vi "r3_Pick&Place_module_chip_second.vi"() -> ()   [LabVIEW 2016]
uses:
  Classes/Controllers/I-O/Copy of NI-DAQ Folder/NI-DAQ.lvclass
  D:/INTT/V1/Classes/Controllers/I-O/Copy of I-O Folder/I-O.lvclass
  Classes/Controllers/Dispenser/Copy of Ultimus V2 Folder/Ultimus V2.lvclass
  <vilib>/Analysis/coordinate.llb/2D Cartesian Coordinate Rotation (Scalar).vi
  <vilib>/Utility/file.llb/Read Delimited Spreadsheet (DBL).vi
  <vilib>/Utility/file.llb/Write Delimited Spreadsheet (DBL).vi
  Classes/Controllers/Motion/Copy of Motion Folder/Motion.lvclass
  Classes/Controllers/Camera/Copy of Controller Folder/Controller.lvclass
  <vilib>/Analysis/NI_AALPro.lvlib
  Classes/Controllers/I-O/Copy of I-O Folder/I-O.lvclass
panel:
  in  "offset":dbl[](array[numeric])
  out "air pressure indecator":i32
  in  "glue deposit group":i32=4
  in  "Ultimus Pressure":i16=20
  in  "Values":bool[](array[boolean])=[FALSE, FALSE]
  out "vacuum on?":bool[](array[boolean])
  out "Array 2":dbl[][](array[numeric])
  out "Measured PickupTool position":dbl[][](array[numeric])
  in  "sampel vacuum":i32[](array[numeric])=[15, 19]
  in  "VacChannel for sample":i32=1
  in  "TrayVaccum":bool
  in  "check height? 2":bool
  in  "check height?":bool
  out "Needle parking position":dbl[](array[numeric])
  out "GlueBox":dbl[][](array[numeric])
  out "appended array":dbl[][](array[numeric])
  in  "chip placement height compensation":dbl=-0.47 format="%#_13g"
  out "Sample on HDI":dbl[][](array[numeric]) format="%#_8g"
  in  "Sensor A/B":bool
  out "Gantry current position":dbl[](array[numeric])
  in  "READ Position":bool
  in  "Needle Height Compenstation\n(glue gap)":dbl=0.34
  in  "Needle Alignment":bool
  in  "Parking position":dbl[](array[numeric])=[625.0, 625.0, 0.0, 0.01]
  in  "GOTO":bool
  in  "Default Pickup Tool Position":dbl[][](array[numeric])=[[153.043, 779.997, 54.962, 0.0365632], [153.043, 779.997, 54.962, 0.0365632]]
  in  "Number of Chips/Sensors \nto be assembled":i32=1
  in  "Default HDI alignment \nmark position":dbl[](array[numeric])=[292.437, 991.477, 79.3487, -0.011805]
  in  "Default HDI size":dbl[](array[numeric])=[24.3371, 231.337, -0.0132064, -0.000194865]
  out "# of tasks excuted":i32
  out "Chips on tray position":dbl[][](array[numeric])
  out "measured HDI size":dbl[](array[numeric])
  in  "Chip tray":dbl[](array[numeric])=[465.031, 710.639, 69.8028, 0.00407755]
  out "Sample position \non HDI":dbl[][](array[numeric])
  in  "Inititalize":bool
  in  "Pick and place":bool
  in  "Deposit Glue":bool
  in  "Measure Pickup Tools":bool
  in  "Measure Samples on tray":bool
  out "default chip and sensor position w.r.t. 1st mark":dbl[][](array[numeric])
  in  "Assembly Type":bool=TRUE
  in  "Stop":bool
  in  "Measure HDI":bool
  out "Measure HDI top-left":dbl[](array[numeric])
  # "Sensor Tray \nVacuum Channel"
  # "Chips"
  # "Sensor 0.3 -> 200 micron glue thickness\nChips 0.34-> 150 micron glue thickness"
  # "Sensors"
  # "Sensor B short"
  # "Sensors B\n(Short)"
  # "Sensors A\n(Long)"
  # "Chips : -0.47-> 60 micron height gap\n               -0.5 -> 90 micron"
  # "Sensor A long"
  # "ACTIONS"
  # "2"
  # "HDI infomation"
  # "chips use channel 0, 2\nsensors use channel 0, 1"
  # "sensor height 69.8471\nchip height 84.693"
  # "Pick and Place"
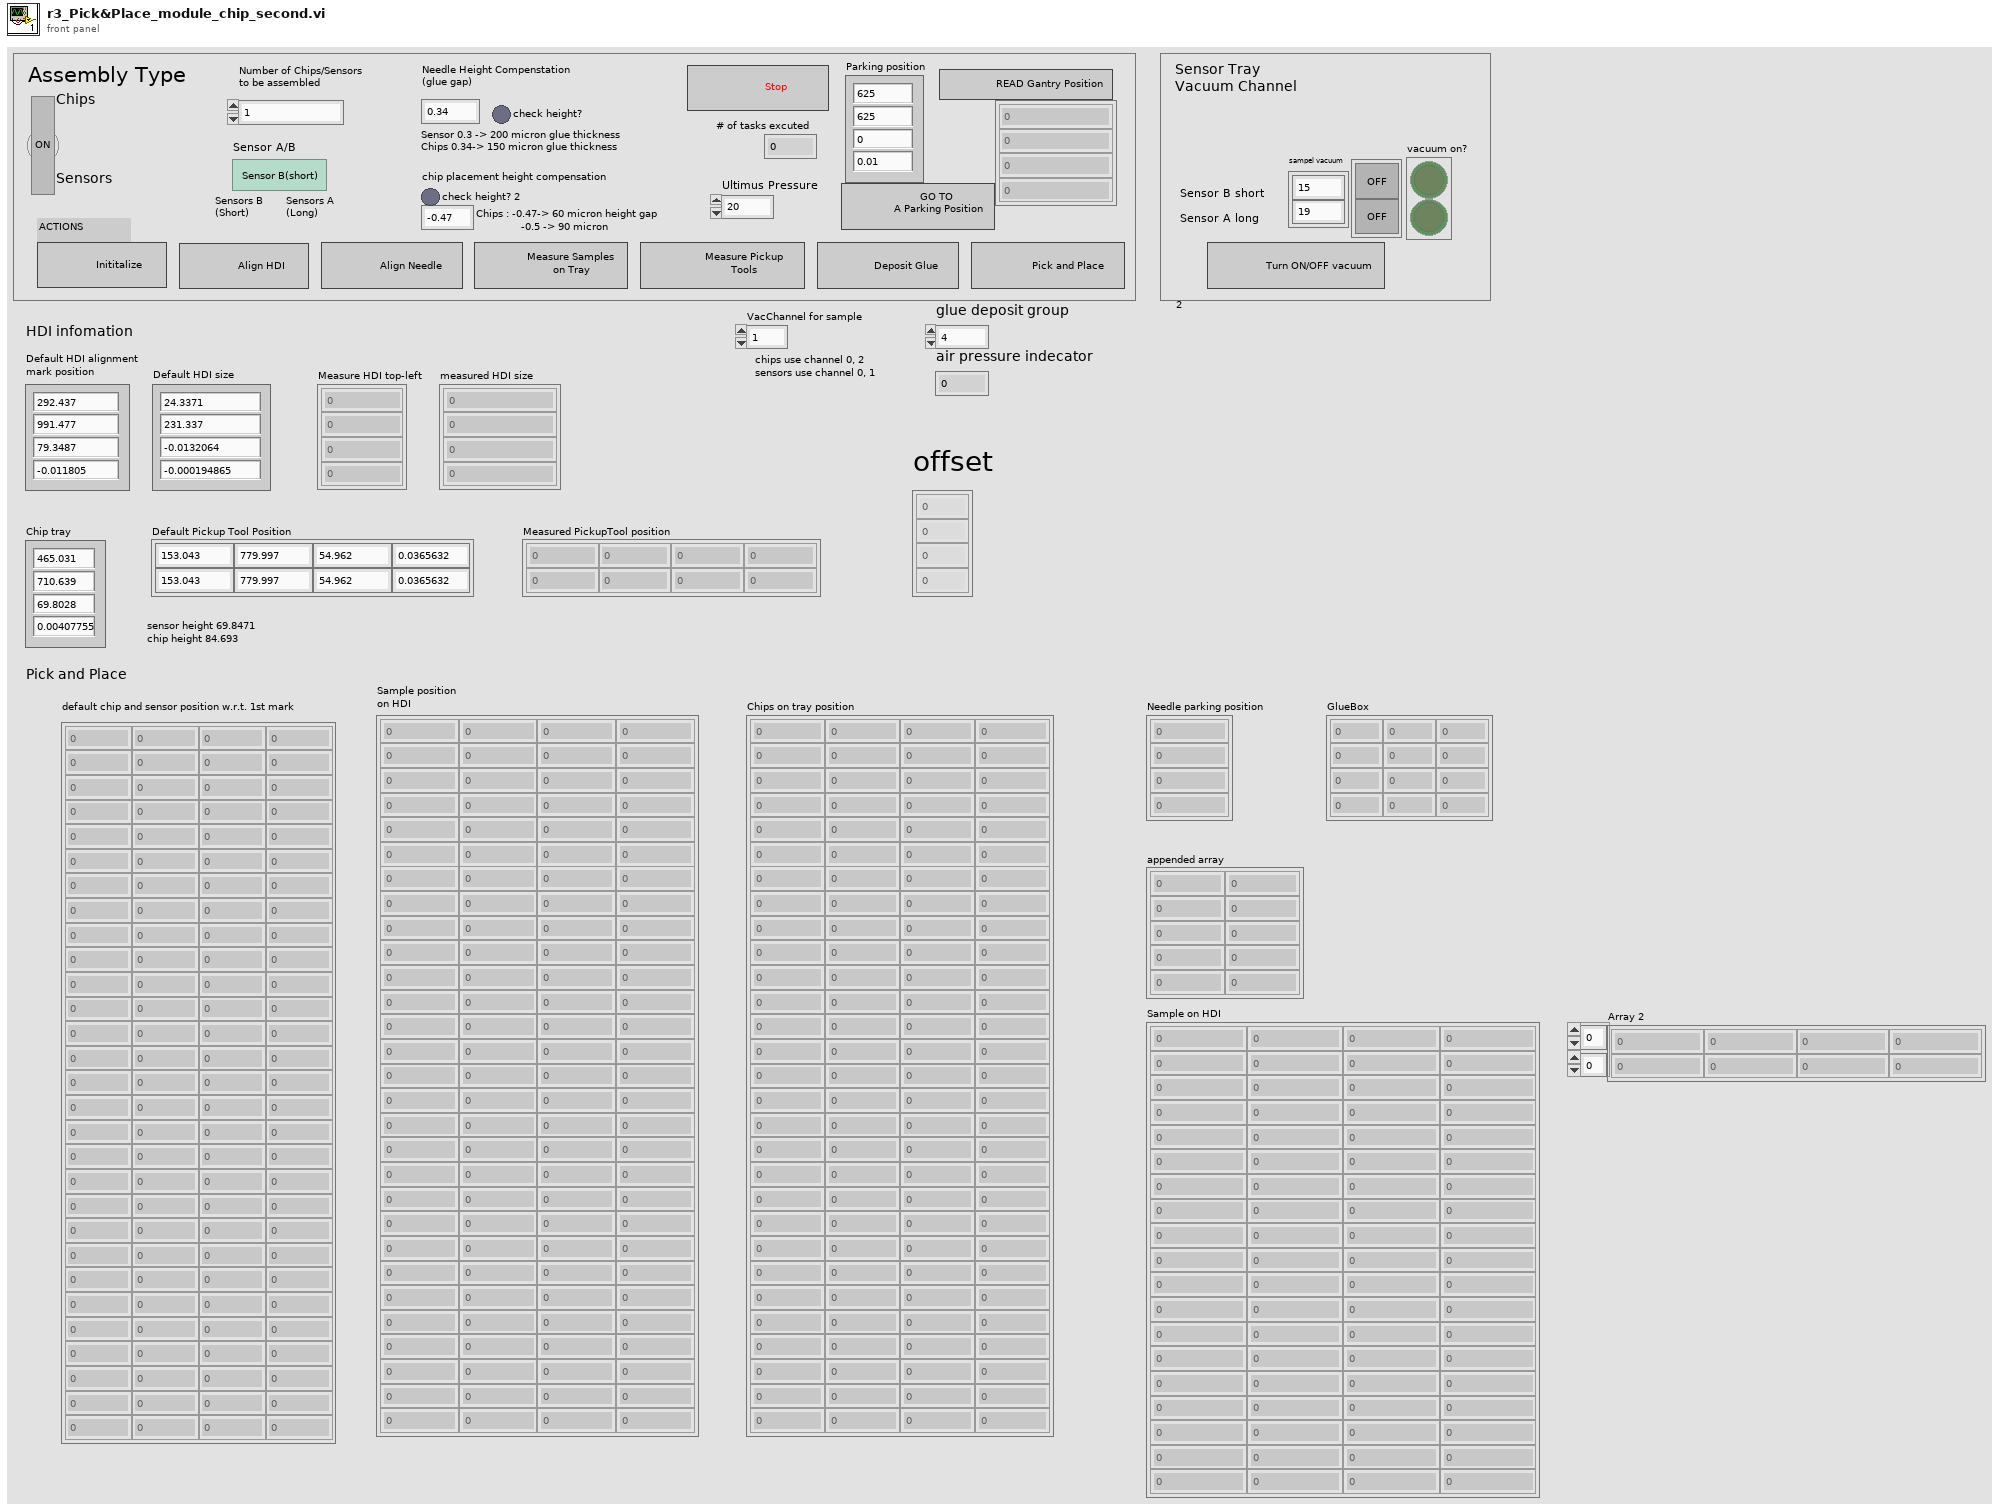
[diagram p1: front panel]
types:
  T1 = typedef "Controller.lvclass/Controllers.ctl" = cluster{"Copy of Motion.lvclass":refnum<class "Motion.lvclass">, "Copy of I-O.lvclass":refnum<class "I-O.lvclass">, "Copy of Dispenser.lvclass":refnum<class "Dispenser.lvclass">}
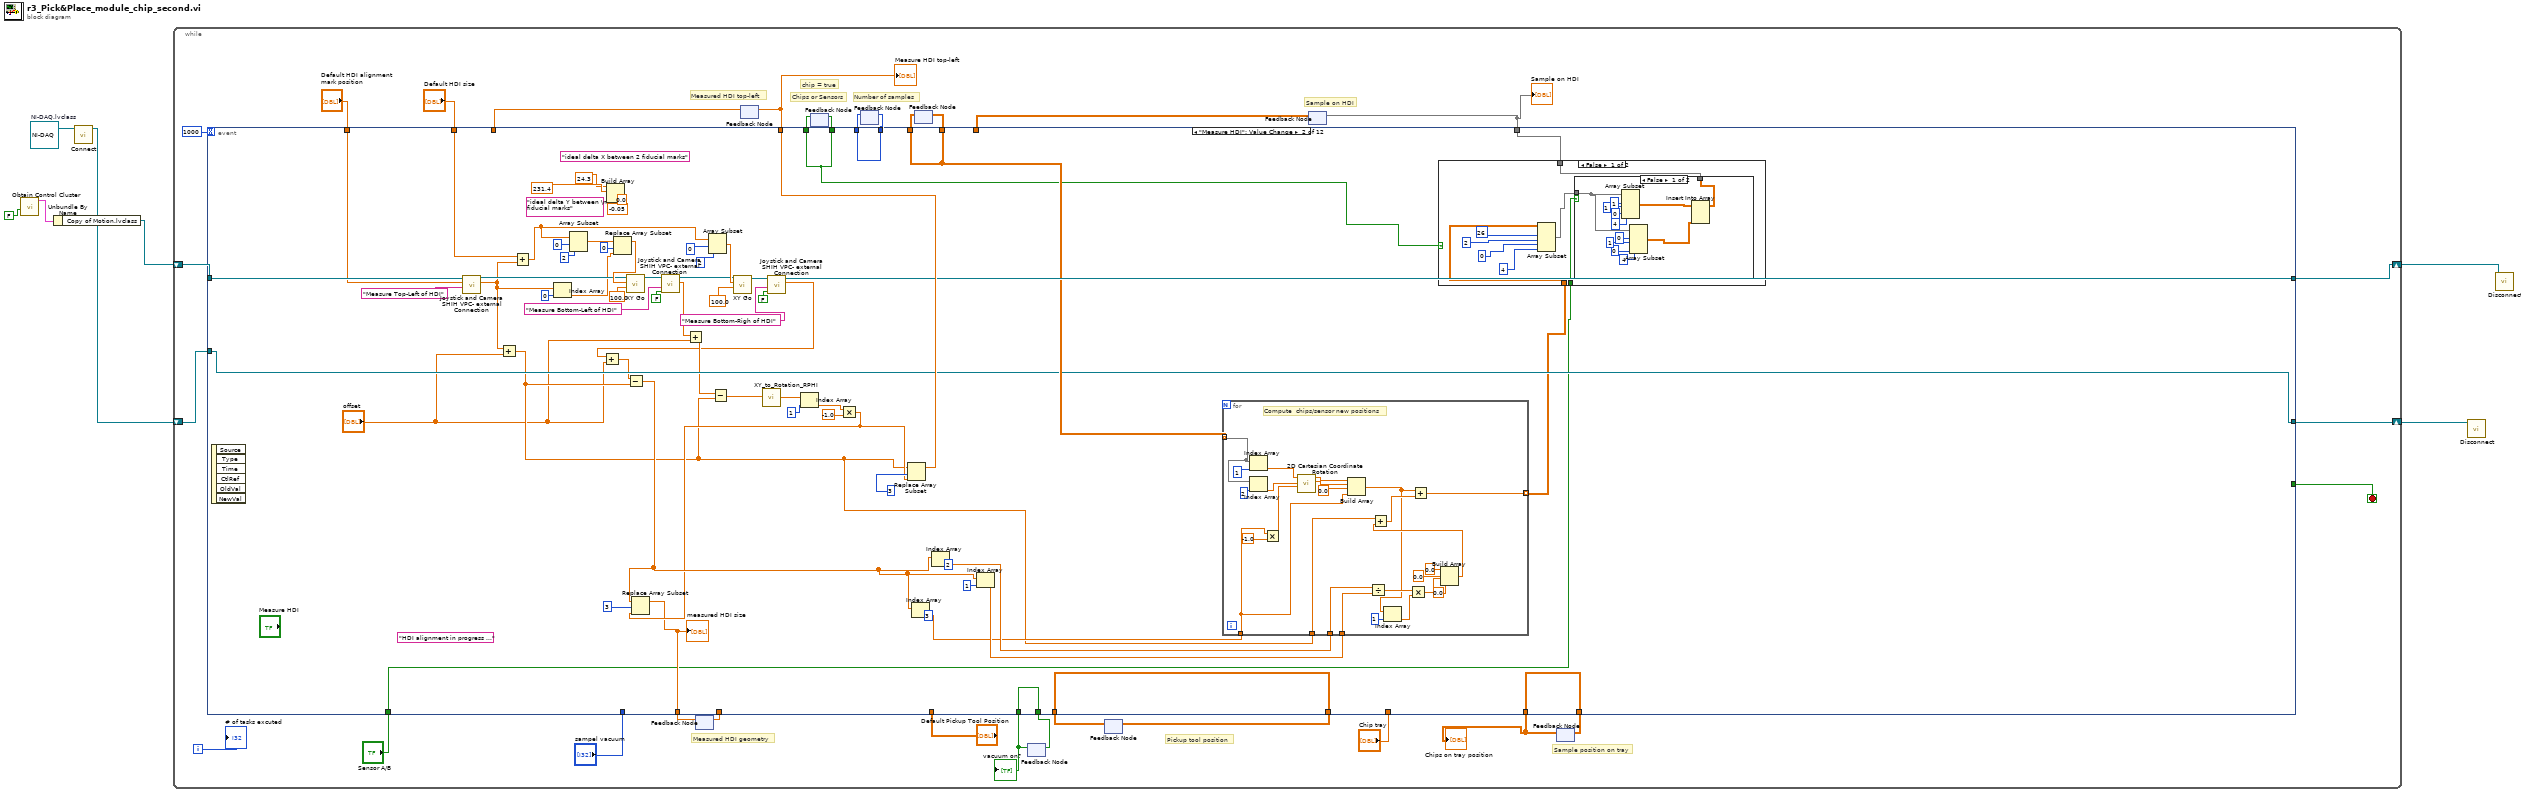
[diagram p0: block diagram]
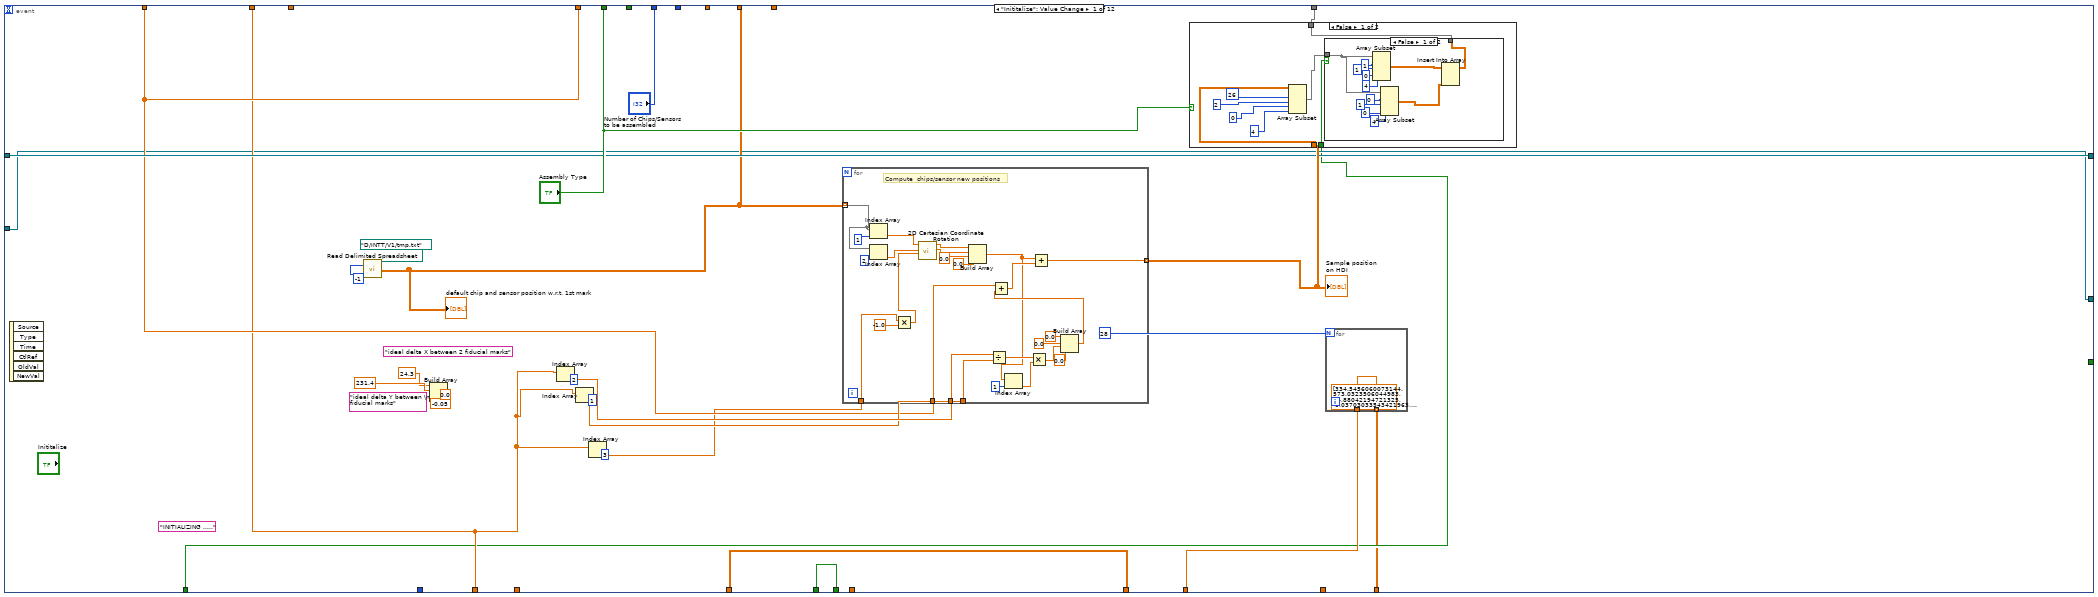
[diagram p2: hidden frame]
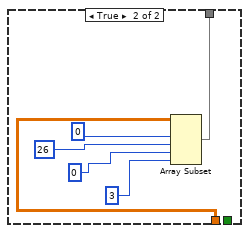
[diagram p4: hidden frame]
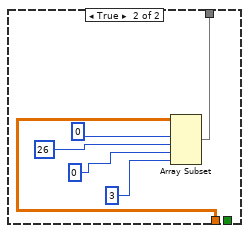
[diagram p6: hidden frame]
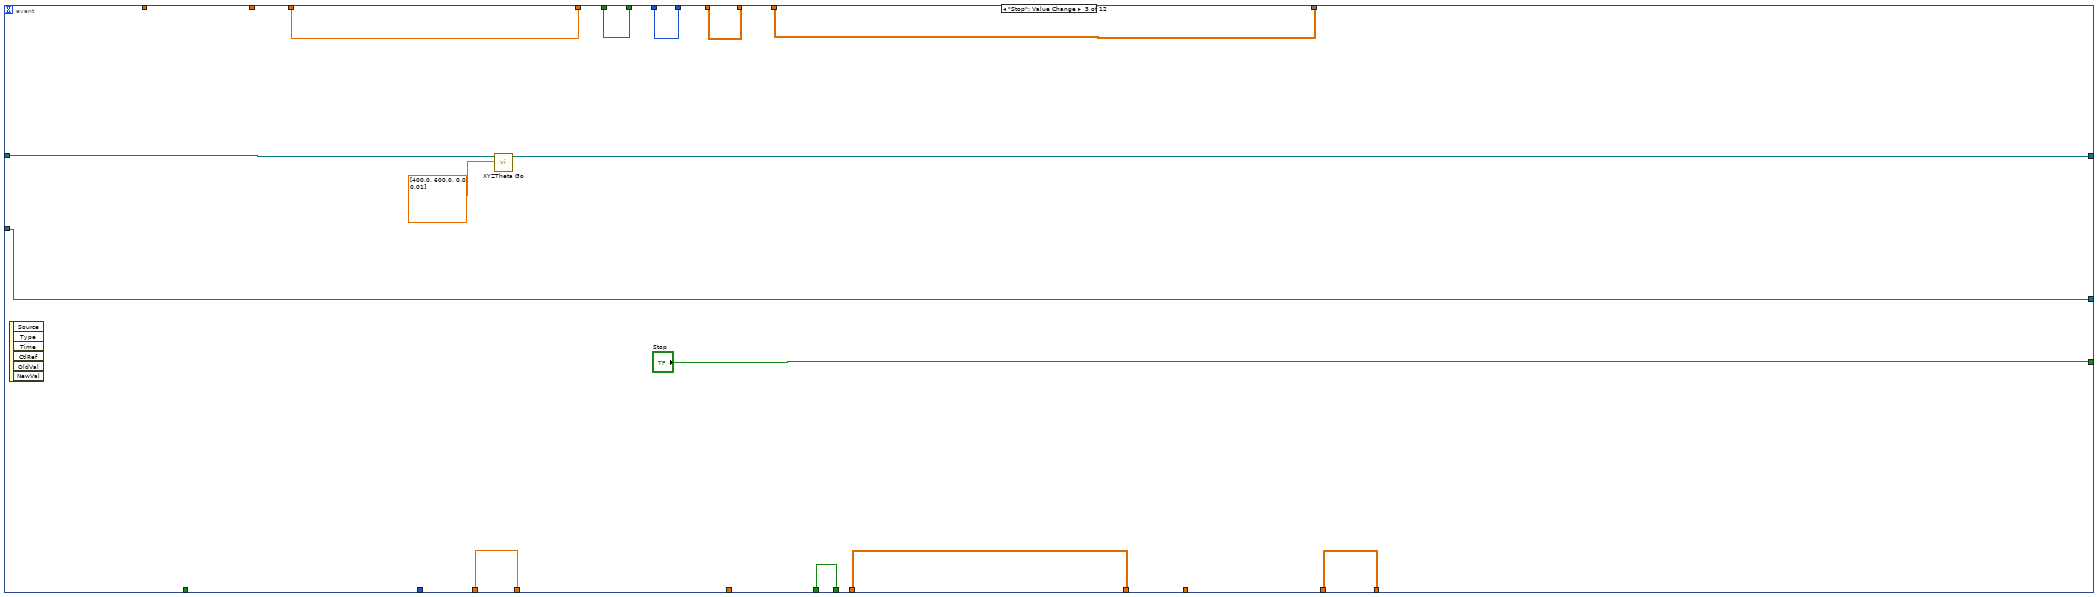
[diagram p7: hidden frame]
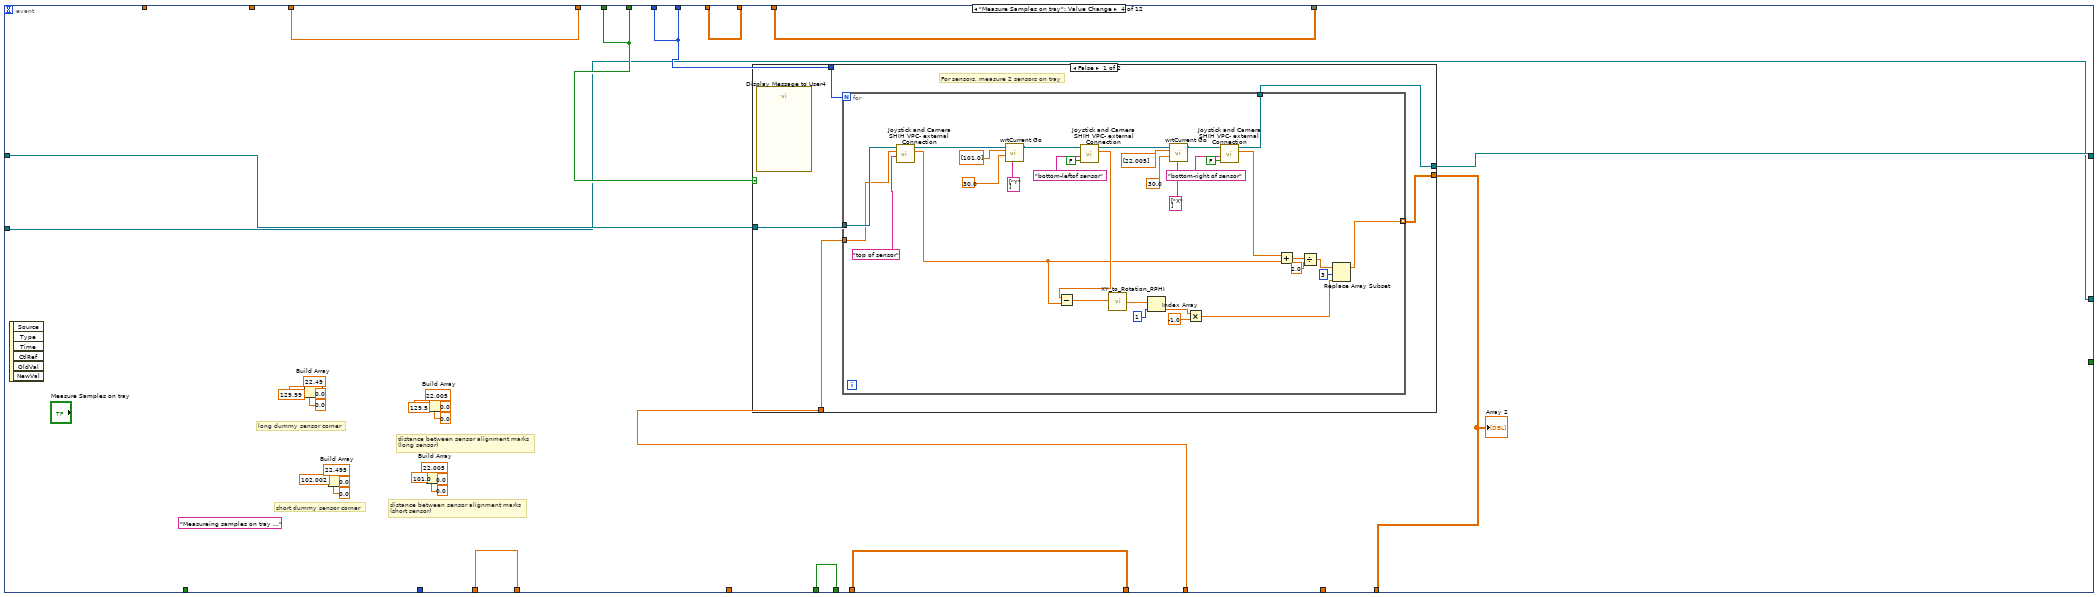
[diagram p8: hidden frame]
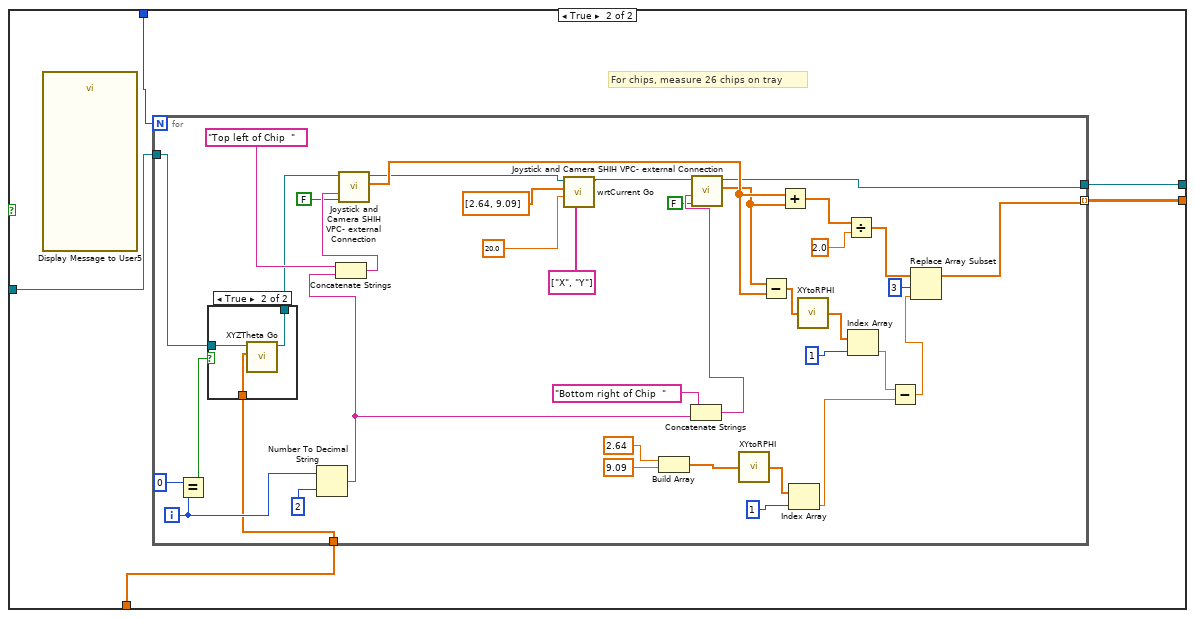
[diagram p9: hidden frame]
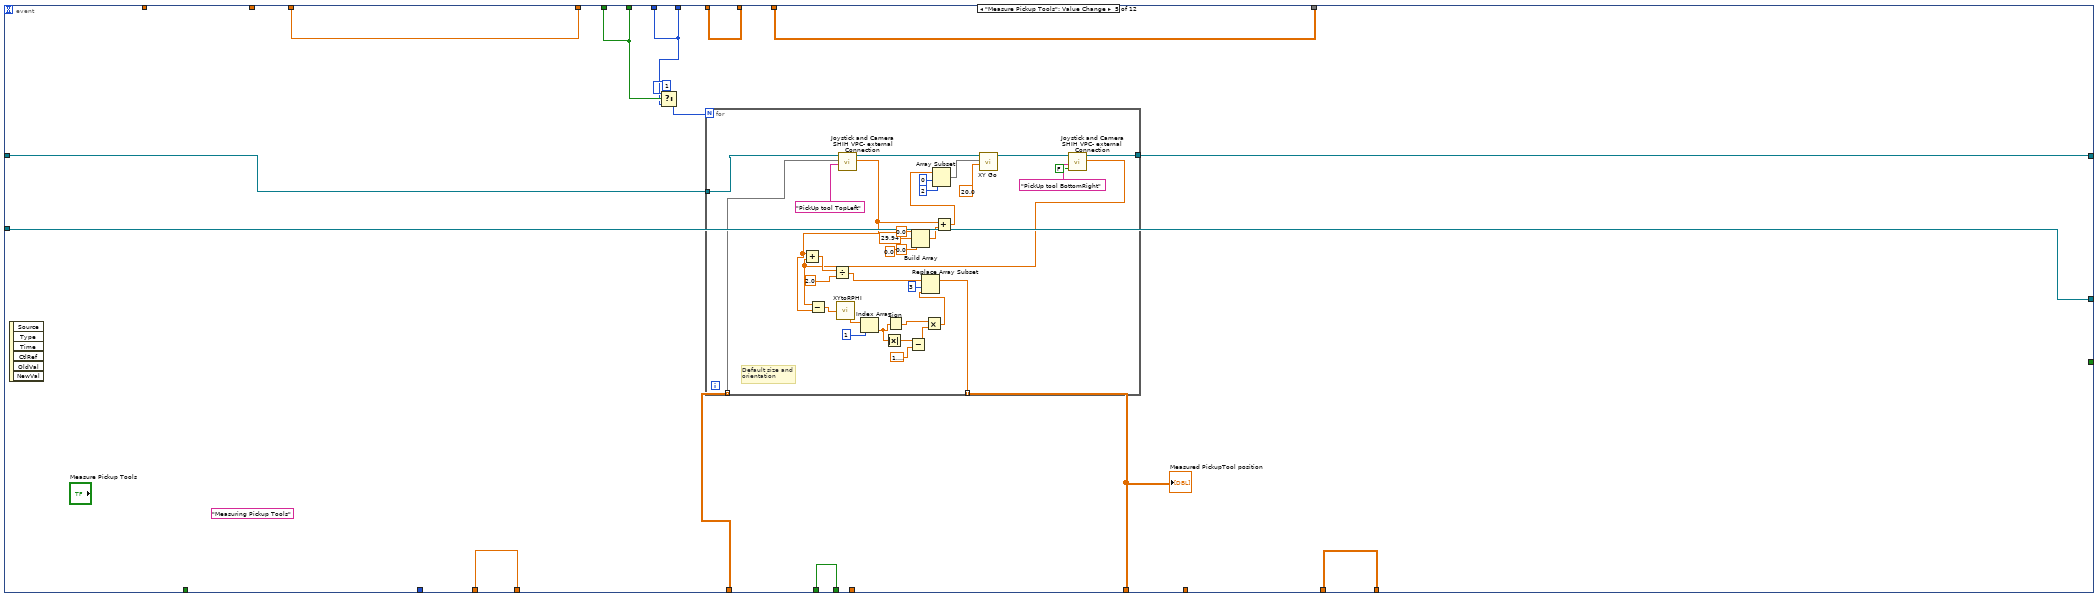
[diagram p11: hidden frame]
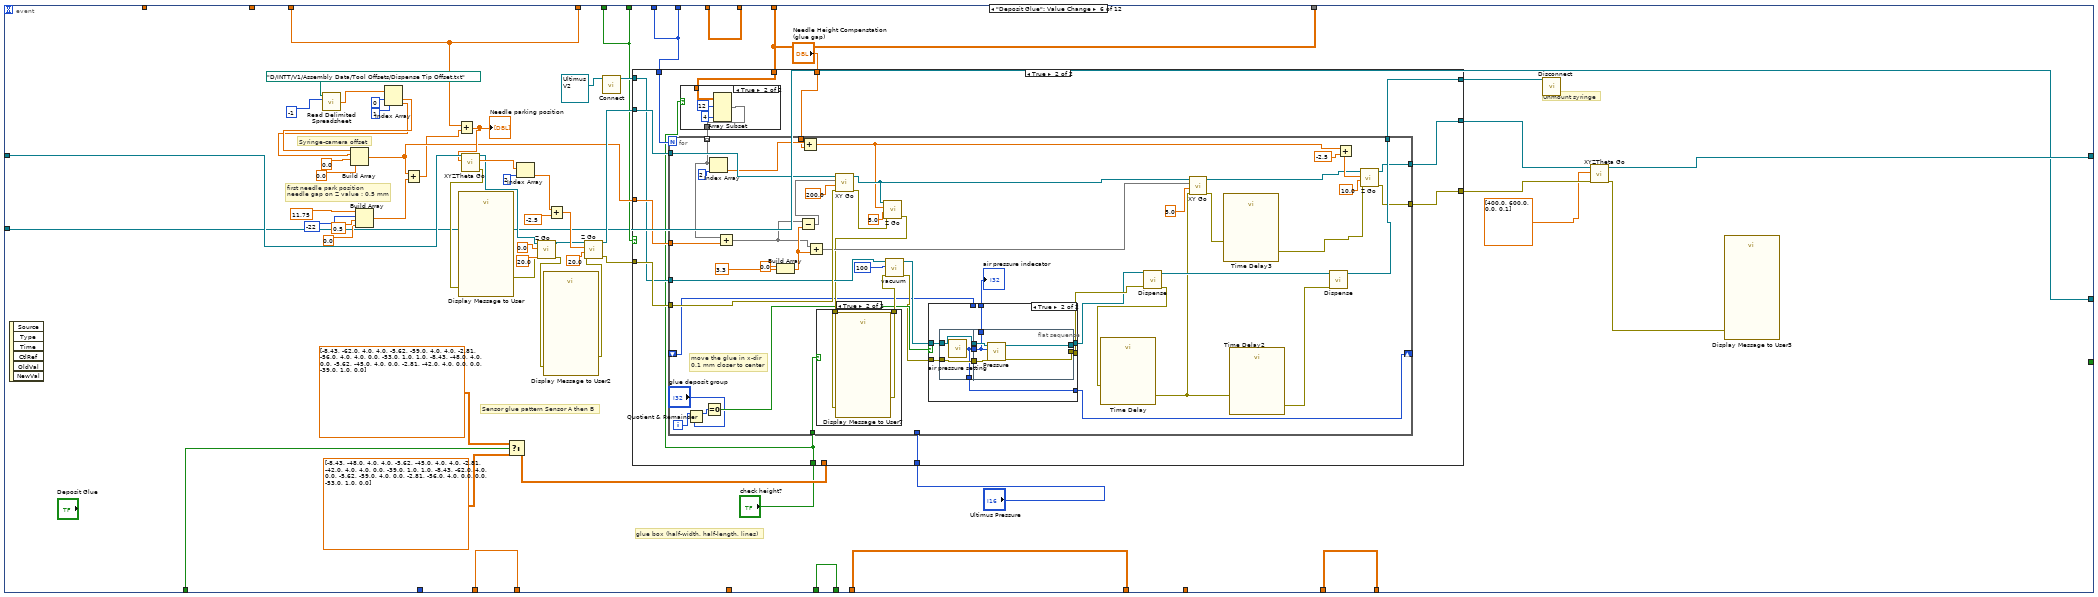
[diagram p12: hidden frame]
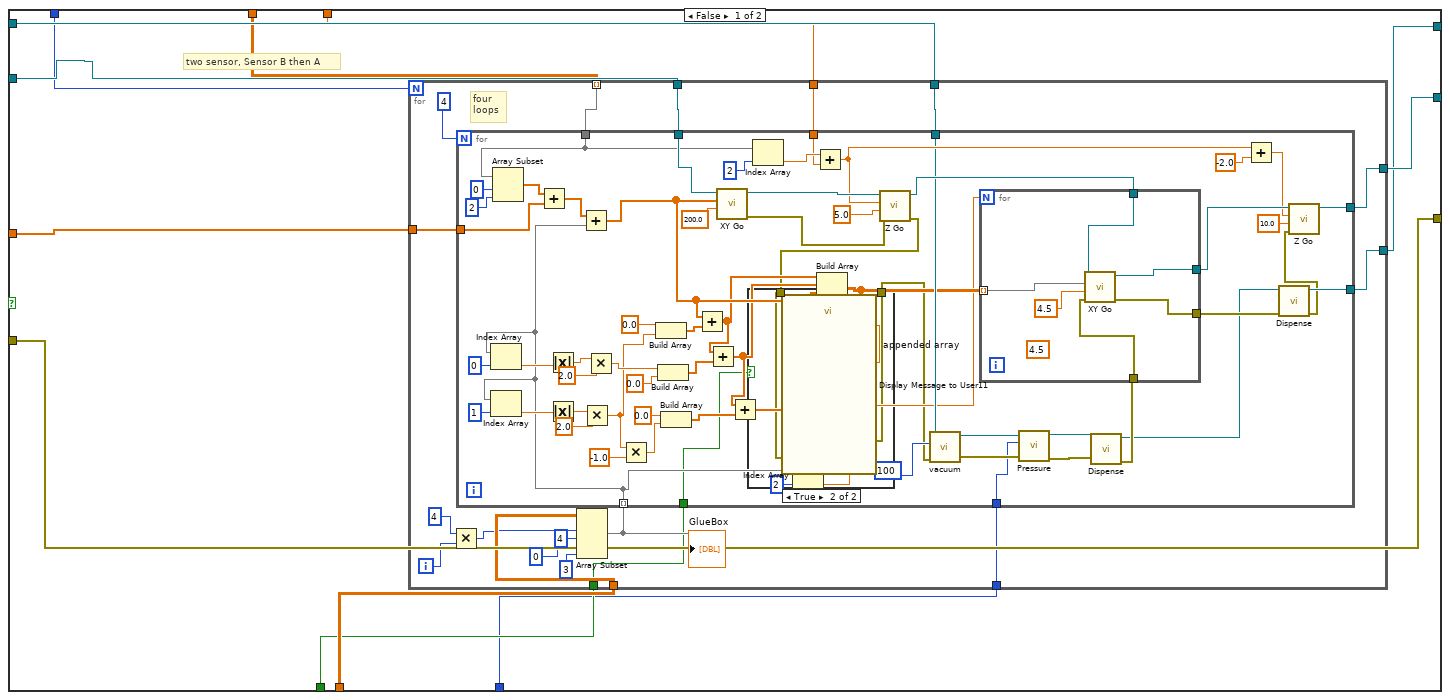
[diagram p13: hidden frame]
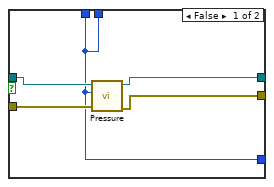
[diagram p16: hidden frame]
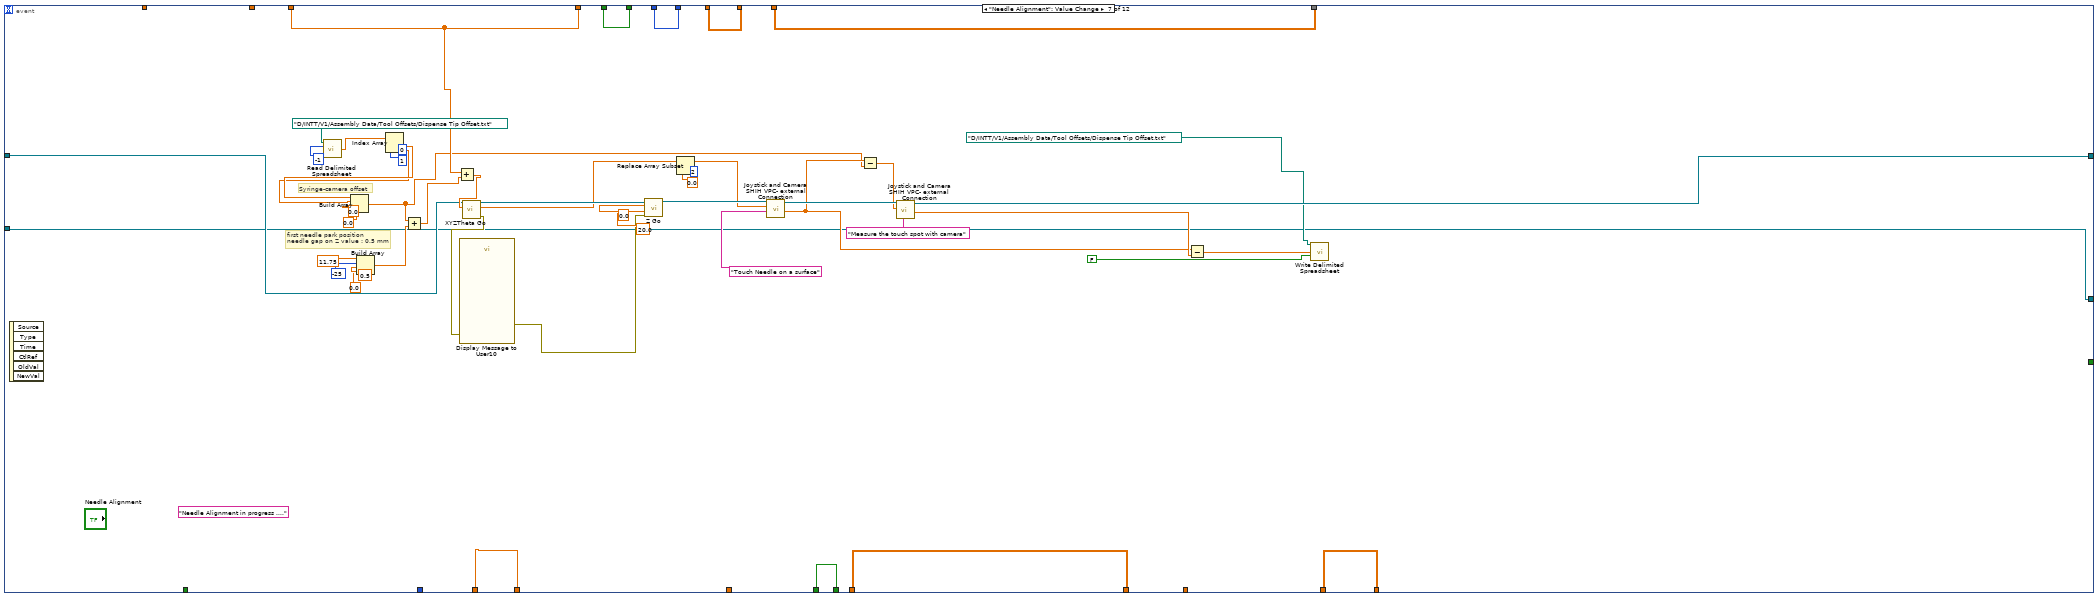
[diagram p18: hidden frame]
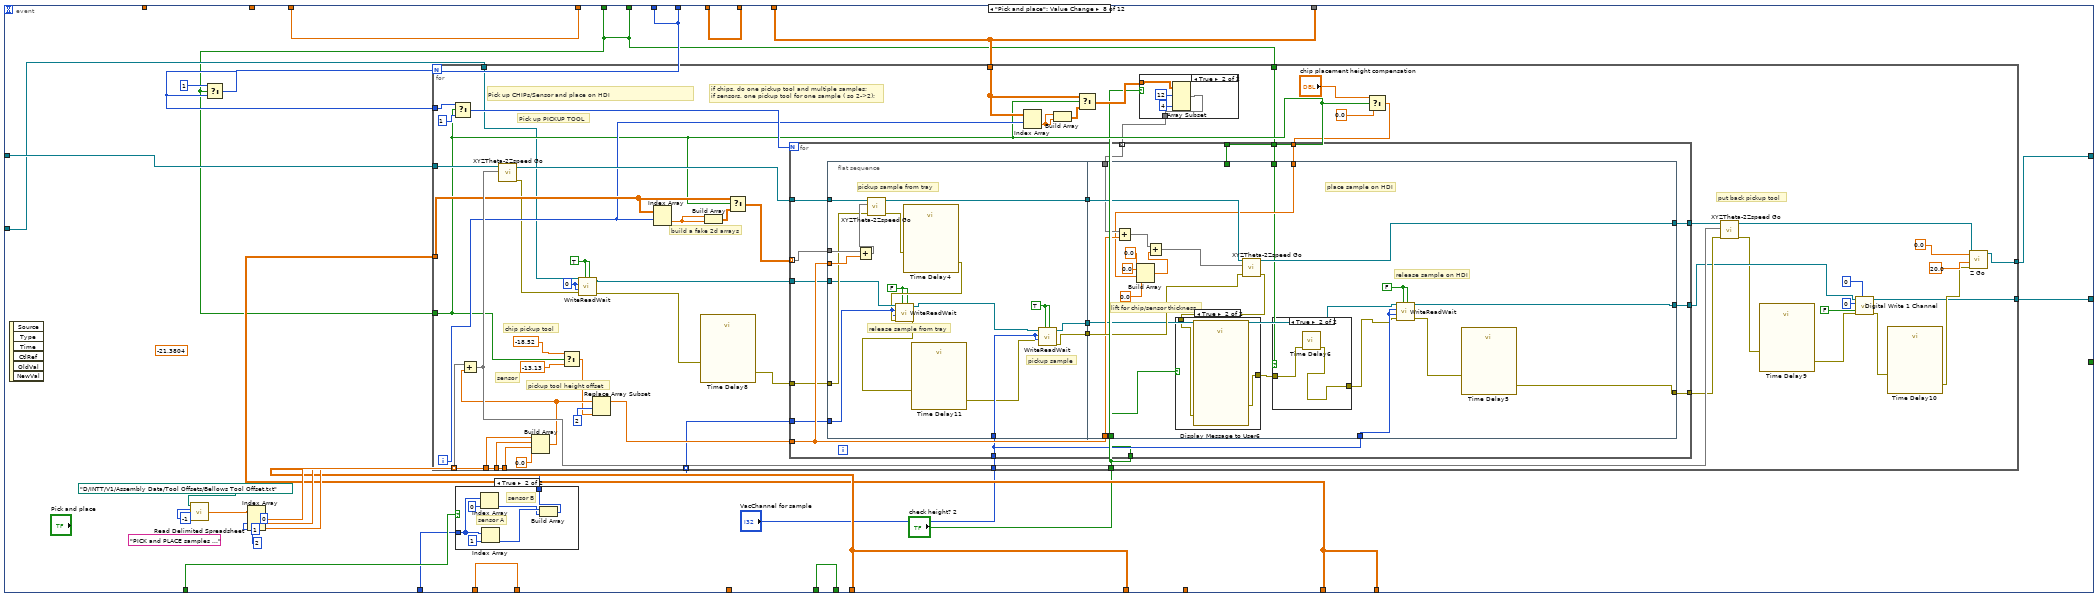
[diagram p19: hidden frame]
diagram:
  w3 = refnum<class "NI-DAQ.lvclass"> refnum  # NI-DAQ.lvclass
  n1 = call "Obtain Control Cluster.vi"("I/O"=FALSE) -> ("Control Out"=w7:T1)  [unwired: 10 in]
  n2 = Unbundle By Name(w7) -> ("Copy of Motion.lvclass"=w5:refnum<class "Motion.lvclass">)
  n3 = call-dynamic "Connect.vi"("NI-DAQ in"=w3) -> ("NI-DAQ out"=w2:refnum<class "NI-DAQ.lvclass">)  [unwired: 9 in, 1 out]
  n4 = while {
    shift-right: [w26] -> w4
    shift-left: w5 -> [w38]
    shift-right: [w13] -> w1
    shift-left: w2 -> [w14]
    i -> [w25]
    stop <- w37 stop-if-true
    # "chip = true"
    # "Pickup tool position"
    # "Chips or Sensors"
    # "Number of samples"
    # "Measured HDI geometry"
    # "Sample position on tray"
    # "Measured HDI top-left"
    # "Sample on HDI"
    n5 = feedback #1() -> (w33:dbl[])  [unwired: 1 in]
    n6 = feedback #2() -> (w35:dbl[])  [unwired: 1 in]
    n7 = feedback #3() -> (w30:bool)  [unwired: 1 in]
    n8 = feedback #4() -> (w24:i32)  [unwired: 1 in]
    n9 = feedback #5() -> (w19:dbl[][])  [unwired: 1 in]
    n10 = feedback #6() -> (w10:bool[])  [unwired: 1 in]
    n11 = feedback #7() -> (w27:dbl[][])  [unwired: 1 in]
    n12 = feedback #8() -> (w32:dbl[][])  [unwired: 1 in]
    n13 = feedback #9() -> (w16:dbl[][])  [unwired: 1 in]
    "Chips on tray position" <- w16
    n14 = event shown="[1] \"Measure HDI\": Value Change" {
      selector: _ -> [_ _ _ _ _ _ _ _ _ _ _ _]
      dyn-events: _ -> [_ _ _ _ _ _ _ _ _ _ _ _]
      timeout: 1000 -> [_ _ _ _ _ _ _ _ _ _ _ _]
      tunnel: w38 -> [w52 w183 w249 w278 w376 w445 w681 w737 w878 w900 w924 w926]
      tunnel: [_ _ "Stop" _ _ _ _ _ _ _ _ _] -> w37
      tunnel: [w49 w181 w242 w272 w367 w426 w689 w721 w887 w894 w920 w937] -> w36
      tunnel: w35 -> [_ _ w242 w272 w367 w426 w689 w721 w887 w894 w920 w937]
      tunnel: ["Assembly Type" w129 w246 w276 w372 w429 w688 w711 w886 w895 w921 w936] -> w31
      tunnel: [w45 w133 w241 w271 w366 w422 w684 w720 w882 w893 w919 w930] -> w34
      tunnel: w33 -> [_ _ w241 w271 w366 w422 w684 w720 w882 w893 w919 w930]
      tunnel: [w40 w130 w243 w273 w369 w428 w685 w726 w883 w898 w923 w933] -> w8
      tunnel: w32 -> [_ _ w243 w273 w369 w428 w685 w726 w883 w898 w923 w933]
      tunnel: w30 -> [_ w129 w246 w276 w372 w429 w688 w711 w886 w895 w921 w936]
      tunnel: w24 -> [_ w172 w245 w275 w371 w427 w687 w723 w885 w896 w916 w935]
      tunnel: [w39 w170 w239 w252 w365 w424 w682 w724 w880 w891 w917 w932] -> w29
      tunnel: w16 -> [_ w170 w239 _ w365 w424 w682 w724 w880 w891 w917 w932]
      tunnel: [w48 w171 w240 w270 w375 w423 w683 w725 w881 w892 w918 w931] -> w28
      tunnel: w27 -> [_ w171 w240 w270 _ w423 w683 w725 w881 w892 w918 w931]
      tunnel: [w52 w180 w247 w277 w374 w430 w673 w727 w877 w899 w924 w926] -> w26
      tunnel: ["Number of Chips/Sensors \nto be assembled" w172 w245 w275 w371 w427 w687 w723 w885 w896 w916 w935] -> w23
      tunnel: "Default HDI alignment \nmark position" -> [w49 w179 _ _ _ _ _ _ _ _ _ _]
      tunnel: "Default HDI size" -> [w45 w178 _ _ _ _ _ _ _ _ _ _]
      tunnel: [w50 w173 w244 w274 w368 w421 w686 w722 w884 w897 w922 w934] -> w20
      tunnel: w19 -> [_ w173 w244 w274 w368 w421 w686 w722 w884 w897 w922 w934]
      tunnel: "Default Pickup Tool Position" -> [w48 _ _ _ w370 _ _ _ _ _ _ _]
      tunnel: "Chip tray" -> [w47 _ _ w269 _ _ _ _ _ _ _ _]
      tunnel: "Sensor A/B" -> [w42 w128 _ _ _ w420 _ w719 _ _ _ _]
      tunnel: w14 -> [w43 w132 w237 w251 w364 w414 w664 w716 w879 w889 w915 w927]
      tunnel: [w43 w132 w237 w251 w364 w414 w664 w717 w879 w889 w901 w925] -> w13
      tunnel: "sampel vacuum" -> [_ _ _ _ _ _ _ w713 _ _ w903 w928]
      tunnel: [w41 w131 w236 w250 w363 w413 w663 w712 w875 w888 w902 w929] -> w11
      tunnel: w10 -> [w41 w131 w236 w250 w363 w413 w663 w712 w875 w888 w902 _]
      event "Inititalize": Value Change {
        (unwired) dbl[][] [[334.5456060073144, 573.0323506044983, 84.88042194721325, -0.03703033543421963], [348.7343172517964, 572.8622513715641, 84.88042161151989, 0.002496633181773955], [362.2570314501057, 572.9994237111084, 84.87348419133077, 0.0034316271147138977], [374.6597880882888, 573.1847541366935, 84.85760352984227, -0.00879928913304795], [388.2847032482186, 573.1649677768512, 84.84172357788742, -0.026054726433181852], [334.1328739355822, 593.938164573938, 84.85715223326392, 0.0033385186776999642], [348.32260344605317, 593.1627350557167, 84.85715229429908, 0.032527677556001944], [361.94845426967004, 593.1988990556995, 84.85715231337257, 0.010856722342177383], [375.3711307391728, 592.862734170051, 84.81179255805122, 0.023593691294119035], [388.0023391138823, 592.7263595201845, 84.81179247794259, -0.025867399820654446], [333.741332819156, 613.4501439838673, 84.86893968673877, 0.012458442710573392], [347.4966613938597, 613.1815273693476, 84.84113487130284, 0.02669962172184226], [360.982501589219, 613.368579091193, 84.84113464623572, -0.018470295852746066], [333.329425210144, 634.0016681075332, 84.84113694649815, -0.011509836209115054], [347.60697621578583, 633.6458142671074, 84.84113655739904, -0.014006699863984284], [362.03055194039933, 633.3683242670324, 84.84113543587804, 0.008503358353721735], [374.6669884842355, 633.6776673973038, 84.82931378598124, -0.012163463061963586], [388.449715198344, 634.0661620162508, 84.81749059876144, -0.029966589814424793], [334.6459562288677, 653.6797245247765, 84.85127519810308, -0.010927379491059153], [348.144539580008, 653.7156084768662, 84.88505952278655, -0.012269636914733706], [361.33508542794345, 653.7223221455167, 84.84332432319749, -0.0225512602477429], [374.2287534347454, 653.8981636020831, 84.87276718319089, 0.0007662059738136051], [387.0483029791335, 653.6404602098912, 84.83290343994173, 0.01982829778783901], [334.77129192493265, 669.5351603609607, 84.8979373024785, 0.03923574774306138], [347.17815774254836, 669.4879675513143, 84.9183079020849, 0.003793410140892961], [361.84116966674696, 669.9123563355322, 84.87756716463502, 0.02903318407151878]] ("Chips on tray position")
        (unwired) "INITIALIZING ....." ("String")
        (unwired) "ideal delta Y between \n2 fiducial marks"
        (unwired) "ideal delta X between 2 fiducial marks"
        n15 = event-data() -> ()  [unwired: 1 in, 6 out]
        n16 = call-poly <vilib>:"Read Delimited Spreadsheet.vi"("file path (dialog if empty)"=path "D:/INTT/V1/tmp.txt", "number of rows (all:-1)"=-1) -> ("all rows"=w50:dbl[][])  [unwired: 8 in, 5 out]
        "default chip and sensor position w.r.t. 1st mark" <- w50
        n17 = Build Array(24.3 ("y"), 231.4 ("y"), 0.0 ("element"), -0.05 ("element")) -> ()  [unwired: 1 out]
        n18 = Index Array(array=w45, index=2) -> (element=w61:dbl)
        n19 = Index Array(array=w45, index=1) -> (element=w60:dbl)
        n20 = Index Array(array=w45, index=3) -> (element=w44:dbl)
        n21 = for {
          tunnel: w50 -> [w112] mode=indexing
          tunnel: w44 -> [w95]
          tunnel: w49 -> [w104]
          tunnel: [w111] -> w54 mode=indexing
          tunnel: w61 -> [w110]
          tunnel: w60 -> [w101]
          # "Compute  chips/sensor new positions"
          n22 = Index Array(array=w112, index=1) -> (element=w116:dbl)
          n23 = Index Array(array=w112, index=2) -> (element=w115:dbl)
          n24 = Multiply(x=w95, y=-1.0) -> (x*y=w96:dbl)
          n25 = call-poly <vilib>:"2D Cartesian Coordinate Rotation.vi"("theta"=w96, "y"=w115, "x"=w116) -> ("y out"=w118:dbl, "x out"=w117:dbl)  [unwired: 6 in, 1 out]
          n26 = Build Array(w117, w118, 0.0 ("element"), 0.0 ("element")) -> (w98:dbl[])
          n27 = Divide(x=w110, y=w101) -> (x/y=w109:dbl)
          n28 = Index Array(array=w98, index=1) -> (element=w99:dbl)
          n29 = Multiply(x=w109, y=w99) -> (x*y=w105:dbl)
          n30 = Build Array(0.0 ("element"), 0.0 ("element"), w105, 0.0 ("element")) -> (w103:dbl[])
          n31 = Add(x=w104, y=w103) -> (x+y=w102:dbl[])
          n32 = Add(x=w98, y=w102) -> (x+y=w111:dbl[])
        }
        "Sample position \non HDI" <- w54
        n33 = case shown="False" "Assembly Type" {
          tunnel: w54 -> [w69 w89]
          tunnel: [w67 w87] -> w40
          tunnel: w42 -> [w66 _]
          frame False {
            n34 = Array Subset(array=w69, index (row)=26 ("index"), length (row)=2 ("length"), index (col)=0, length (col)=4 ("length")) -> (w68:dbl[][])
            n35 = case shown="False" w66 {
              tunnel: w68 -> [w77 w86]
              tunnel: [w74 w86] -> w67
              frame False {
                n36 = Array Subset(array=w77, index (row)=1 ("index"), length (row)=1 ("length"), index (col)=0 ("index"), length (col)=4 ("length")) -> (w76:dbl[][])
                n37 = Array Subset(array=w77, index (row)=0 ("index"), length (row)=1 ("length"), index (col)=0 ("index"), length (col)=4 ("length")) -> (w75:dbl[][])
                n38 = Insert Into Array(array=w76, new element=w75) -> (w74:dbl[][])  [unwired: 2 in]
              }
              frame True {
              }
            }
          }
          frame True {
            n39 = Array Subset(array=w89, index (row)=0 ("index"), length (row)=26 ("length"), index (col)=0, length (col)=3 ("length")) -> (w87:dbl[][])
          }
        }
        n40 = for {
          N: 28 -> [_]
          tunnel: w47 -> [w93]
          tunnel: [w93] -> w39 mode=indexing
        }
      }
      event "Measure HDI": Value Change {
        (unwired) "ideal delta Y between \n2 fiducial marks"
        (unwired) "ideal delta X between 2 fiducial marks"
        (unwired) "HDI alignment in progress ..." ("String")
        n41 = event-data() -> ()  [unwired: 1 in, 6 out]
        n42 = call "Joystick and Camera SHIH VPC- external Connection.vi"("Motion in"=w183, "XYZTheta"=w179, "Measurement Point"="Measure Top-Left of HDI") -> ("Motion out"=w148:refnum<class "Motion.lvclass">, "Sum"=w126:dbl[])  [unwired: 4 in, 2 out]
        n43 = Add(x=w126, y="offset") -> (x+y=w125:dbl[])
        n44 = Add(x=w178, y=w126) -> (x+y=w152:dbl[])
        n45 = Index Array(array=w126, index=0) -> (element=w139:dbl)
        n46 = Array Subset(array=w152, index=0, length=2) -> (w151:dbl[])
        n47 = Build Array(24.3 ("y"), 231.4 ("y"), 0.0 ("element"), -0.05 ("element")) -> ()  [unwired: 1 out]
        n48 = Replace Array Subset(array=w151, new element=w139, index=0) -> (w149:dbl[])
        n49 = call-dynamic "XY Go.vi"("Speed"=100.0, "XY"=w149, "Motion in"=w148) -> ("Motion out"=w156:refnum<class "Motion.lvclass">)  [unwired: 7 in, 1 out]
        n50 = call "Joystick and Camera SHIH VPC- external Connection.vi"("Motion in"=w156, "Measurement Point"="Measure Bottom-Left of HDI", "Inital GO"=FALSE) -> ("Motion out"=w147:refnum<class "Motion.lvclass">, "Sum"=w124:dbl[])  [unwired: 4 in, 2 out]
        n51 = Add(x=w124, y="offset") -> (x+y=w123:dbl[])
        n52 = Array Subset(array=w152, index=0, length=2) -> (w162:dbl[])
        n53 = Subtract(x=w123, y=w125) -> (x-y=w146:dbl[])
        n54 = call-dynamic "XY Go.vi"("Speed"=100.0, "XY"=w162, "Motion in"=w147) -> ("Motion out"=w166:refnum<class "Motion.lvclass">)  [unwired: 7 in, 1 out]
        n55 = call "XY_to_Rotation_RPHI.vi"("X-Y"=w146) -> ("r-phi"=w142:dbl[])
        n56 = call "Joystick and Camera SHIH VPC- external Connection.vi"("Motion in"=w166, "Measurement Point"="Measure Bottom-Righ of HDI", "Inital GO"=FALSE) -> ("Motion out"=w180:refnum<class "Motion.lvclass">, "Sum"=w122:dbl[])  [unwired: 4 in, 2 out]
        n57 = Add(x=w122, y="offset") -> (x+y=w121:dbl[])
        n58 = Subtract(x=w121, y=w125) -> (x-y=w136:dbl[])
        n59 = Index Array(array=w142, index=1) -> (element=w137:dbl)
        n60 = Multiply(x=w137, y=-1.0) -> (x*y=w134:dbl)
        n61 = Replace Array Subset(array=w136, new element=w134, index=3) -> (w133:dbl[])
        "measured HDI size" <- w133
        n62 = Replace Array Subset(array=w125, new element=w134, index=3) -> (w181:dbl[])
        n63 = Index Array(array=w136, index=3) -> (element=w168:dbl)
        n64 = Index Array(array=w136, index=2) -> (element=w175:dbl)
        n65 = Index Array(array=w136, index=1) -> (element=w174:dbl)
        n66 = for {
          tunnel: w173 -> [w228] mode=indexing
          tunnel: w168 -> [w213]
          tunnel: w125 -> [w221]
          tunnel: w175 -> [w227]
          tunnel: w174 -> [w218]
          tunnel: [w211] -> w127 mode=indexing
          # "Compute  chips/sensor new positions"
          n67 = Index Array(array=w228, index=1) -> (element=w232:dbl)
          n68 = Index Array(array=w228, index=2) -> (element=w231:dbl)
          n69 = Multiply(x=w213, y=-1.0) -> (x*y=w212:dbl)
          n70 = call-poly <vilib>:"2D Cartesian Coordinate Rotation.vi"("theta"=w212, "y"=w231, "x"=w232) -> ("y out"=w234:dbl, "x out"=w233:dbl)  [unwired: 6 in, 1 out]
          n71 = Build Array(w233, w234, 0.0 ("element"), w213) -> (w215:dbl[])
          n72 = Divide(x=w227, y=w218) -> (x/y=w226:dbl)
          n73 = Index Array(array=w215, index=1) -> (element=w216:dbl)
          n74 = Multiply(x=w226, y=w216) -> (x*y=w222:dbl)
          n75 = Build Array(0.0 ("element"), 0.0 ("element"), w222, 0.0 ("element")) -> (w220:dbl[])
          n76 = Add(x=w221, y=w220) -> (x+y=w219:dbl[])
          n77 = Add(x=w215, y=w219) -> (x+y=w211:dbl[])
        }
        n78 = case shown="False" w129 {
          tunnel: w127 -> [w187 w207]
          tunnel: [w185 w205] -> w130
          tunnel: w128 -> [w184 _]
          frame False {
            n79 = Array Subset(array=w187, index (row)=26 ("index"), length (row)=2 ("length"), index (col)=0, length (col)=4 ("length")) -> (w186:dbl[][])
            n80 = case shown="False" w184 {
              tunnel: w186 -> [w195 w204]
              tunnel: [w192 w204] -> w185
              frame False {
                n81 = Array Subset(array=w195, index (row)=1 ("index"), length (row)=1 ("length"), index (col)=0 ("index"), length (col)=4 ("length")) -> (w194:dbl[][])
                n82 = Array Subset(array=w195, index (row)=0 ("index"), length (row)=1 ("length"), index (col)=0 ("index"), length (col)=4 ("length")) -> (w193:dbl[][])
                n83 = Insert Into Array(array=w194, new element=w193) -> (w192:dbl[][])  [unwired: 2 in]
              }
              frame True {
              }
            }
          }
          frame True {
            n84 = Array Subset(array=w207, index (row)=0 ("index"), length (row)=26 ("length"), index (col)=0, length (col)=3 ("length")) -> (w205:dbl[][])
          }
        }
      }
      event "Stop": Value Change {
        n85 = event-data() -> ()  [unwired: 1 in, 6 out]
        n86 = call "XYZTheta Go.vi"("XYZTheta In"=dbl[] [400.0, 600.0, 0.0, 0.01], "Motion in"=w249) -> ("Motion out"=w247:refnum<class "Motion.lvclass">)  [unwired: 7 in, 2 out]
      }
      event "Measure Samples on tray": Value Change {
        (unwired) "Measureing samples on tray ..." ("String")
        # "long dummy sensor corner"
        # "short dummy sensor corner"
        # "distance between sensor alignment marks\n(short sensor)"
        # "distance between sensor alignment marks\n(long sensor)"
        n87 = event-data() -> ()  [unwired: 1 in, 6 out]
        n88 = Build Array(22.49 ("element"), 129.99 ("element"), 0.0 ("element"), 0.0 ("element")) -> ()  [unwired: 1 out]
        n89 = Build Array(22.495 ("element"), 102.002 ("element"), 0.0 ("element"), 0.0 ("element")) -> ()  [unwired: 1 out]
        n90 = Build Array(22.005 ("element"), 101.0 ("element"), 0.0 ("element"), 0.0 ("element")) -> ()  [unwired: 1 out]
        n91 = Build Array(22.005 ("element"), 129.5 ("element"), 0.0 ("element"), 0.0 ("element")) -> ()  [unwired: 1 out]
        n92 = case shown="False" w276 {
          tunnel: [w280 w320] -> w252
          tunnel: w278 -> [w283 w319]
          tunnel: [w279 w318] -> w277
          tunnel: w275 -> [w282 w317]
          tunnel: w269 -> [w281 w316]
          frame False {
            # "For sensors, measure 2 sensors on tray"
            n93 = call "Display Message to User4"() -> ()  [unwired: 10 in, 2 out]
            n94 = for {
              N: w282 -> [_]
              tunnel: w283 -> [w315]
              tunnel: [w312] -> w279
              tunnel: [w306] -> w280 mode=indexing
              tunnel: w281 -> [w305]
              n95 = call "Joystick and Camera SHIH VPC- external Connection.vi"("Motion in"=w315, "XYZTheta"=w305, "Measurement Point"="top of sensor") -> ("Motion out"=w287:refnum<class "Motion.lvclass">, "Sum"=w294:dbl[])  [unwired: 4 in, 2 out]
              n96 = call-dynamic "wrtCurrent Go.vi"("axis names"=string[] ["Y"], "Speed"=30.0, "distances"=dbl[] [101.0], "Motion in"=w287) -> ("Motion out"=w286:refnum<class "Motion.lvclass">)  [unwired: 6 in, 1 out]
              n97 = call "Joystick and Camera SHIH VPC- external Connection.vi"("Motion in"=w286, "Measurement Point"="bottom-leftof sensor", "Inital GO"=FALSE) -> ("Motion out"=w292:refnum<class "Motion.lvclass">, "Sum"=w296:dbl[])  [unwired: 4 in, 2 out]
              n98 = Subtract(x=w296, y=w294) -> (x-y=w301:dbl[])
              n99 = call "XY_to_Rotation_RPHI.vi"("X-Y"=w301) -> ("r-phi"=w300:dbl[])
              n100 = Index Array(array=w300, index=1) -> (element=w297:dbl)
              n101 = call-dynamic "wrtCurrent Go.vi"("axis names"=string[] ["X"], "Speed"=30.0, "distances"=dbl[] [22.005], "Motion in"=w292) -> ("Motion out"=w293:refnum<class "Motion.lvclass">)  [unwired: 6 in, 1 out]
              n102 = Multiply(x=w297, y=-1.0) -> (x*y=w295:dbl)
              n103 = call "Joystick and Camera SHIH VPC- external Connection.vi"("Motion in"=w293, "Measurement Point"="bottom-right of sensor", "Inital GO"=FALSE) -> ("Motion out"=w312:refnum<class "Motion.lvclass">, "Sum"=w309:dbl[])  [unwired: 4 in, 2 out]
              n104 = Add(x=w309, y=w294) -> (x+y=w310:dbl[])
              n105 = Divide(x=w310, y=2.0) -> (x/y=w308:dbl[])
              n106 = Replace Array Subset(array=w308, new element=w295, index=3) -> (w306:dbl[])
            }
          }
          frame True {
            # "For chips, measure 26 chips on tray"
            n107 = call "Display Message to User5"() -> ()  [unwired: 10 in, 2 out]
            n108 = for {
              N: w317 -> [_]
              tunnel: [w347] -> w320 mode=indexing
              tunnel: w319 -> [w331]
              tunnel: [w327] -> w318
              tunnel: w316 -> [w332]
              i -> [w335]
              n109 = Equal?(x=0, y=w335) -> (x = y?=w333:bool)
              n110 = case shown="True" w333 {
                tunnel: w332 -> [_ w362]
                tunnel: w331 -> [w359 w361]
                tunnel: [w359 w360] -> w330
                frame False {
                }
                frame True {
                  n111 = call "XYZTheta Go.vi"("XYZTheta In"=w362, "Motion in"=w361) -> ("Motion out"=w360:refnum<class "Motion.lvclass">)  [unwired: 7 in, 2 out]
                }
              }
              n112 = Number To Decimal String(number=w335, width (-)=i16 2) -> (decimal integer string=w351:string)
              n113 = Concatenate Strings("Top left of Chip  " ("string"), w351) -> (w345:string)
              n114 = call "Joystick and Camera SHIH VPC- external Connection.vi"("Motion in"=w330, "Measurement Point"=w345, "Inital GO"=FALSE) -> ("Motion out"=w324:refnum<class "Motion.lvclass">, "Sum"=w350:dbl[])  [unwired: 4 in, 2 out]
              n115 = call-dynamic "wrtCurrent Go.vi"("axis names"=string[] ["X", "Y"], "Speed"=20.0, "distances"=dbl[] [2.64, 9.09], "Motion in"=w324) -> ("Motion out"=w325:refnum<class "Motion.lvclass">)  [unwired: 6 in, 1 out]
              n116 = Build Array(2.64 ("element"), 9.09 ("element")) -> (w340:dbl[])
              n117 = Concatenate Strings("Bottom right of Chip  " ("string"), w351) -> (w329:string)
              n118 = call "Joystick and Camera SHIH VPC- external Connection.vi"("Motion in"=w325, "Measurement Point"=w329, "Inital GO"=FALSE) -> ("Motion out"=w327:refnum<class "Motion.lvclass">, "Sum"=w326:dbl[])  [unwired: 4 in, 2 out]
              n119 = call "XYtoRPHI.vi"("X-Y"=w340) -> ("r-phi"=w342:dbl[])
              n120 = Subtract(x=w326, y=w350) -> (x-y=w343:dbl[])
              n121 = Add(x=w350, y=w326) -> (x+y=w355:dbl[])
              n122 = Index Array(array=w342, index=1) -> (element=w337:dbl)
              n123 = call "XYtoRPHI.vi"("X-Y"=w343) -> ("r-phi"=w354:dbl[])
              n124 = Divide(x=w355, y=2.0) -> (x/y=w349:dbl[])
              n125 = Index Array(array=w354, index=1) -> (element=w338:dbl)
              n126 = Subtract(x=w338, y=w337) -> (x-y=w339:dbl)
              n127 = Replace Array Subset(array=w349, new element=w339, index=3) -> (w347:dbl[])
            }
          }
        }
        "Array 2" <- w252
      }
      event "Measure Pickup Tools": Value Change {
        (unwired) "Measuring Pickup Tools" ("String")
        n128 = event-data() -> ()  [unwired: 1 in, 6 out]
        n129 = Select(t=i8 1, s=w372, f=w371) -> (s? t:f=w373:i32)
        n130 = for {
          N: w373 -> [_]
          tunnel: [w401] -> w375 mode=indexing
          tunnel: w376 -> [w405]
          tunnel: [w387] -> w374
          tunnel: w370 -> [w386] mode=indexing
          # "Default size and\norientation"
          n131 = call "Joystick and Camera SHIH VPC- external Connection.vi"("Motion in"=w405, "XYZTheta"=w386, "Measurement Point"="PickUp tool TopLeft") -> ("Motion out"=w381:refnum<class "Motion.lvclass">, "Sum"=w404:dbl[])  [unwired: 4 in, 2 out]
          n132 = Build Array(0.0 ("element"), 29.94 ("element"), 0.0 ("element"), 0.0 ("element")) -> (w392:dbl[])
          n133 = Add(x=w404, y=w392) -> (x+y=w378:dbl[])
          n134 = Array Subset(array=w378, index=0, length=2) -> (w379:dbl[])
          n135 = call-dynamic "XY Go.vi"("Speed"=20.0, "XY"=w379, "Motion in"=w381) -> ("Motion out"=w380:refnum<class "Motion.lvclass">)  [unwired: 7 in, 1 out]
          n136 = call "Joystick and Camera SHIH VPC- external Connection.vi"("Motion in"=w380, "Measurement Point"="PickUp tool BottomRight", "Inital GO"=FALSE) -> ("Motion out"=w387:refnum<class "Motion.lvclass">, "Sum"=w403:dbl[])  [unwired: 4 in, 2 out]
          n137 = Add(x=w404, y=w403) -> (x+y=w410:dbl[])
          n138 = Subtract(x=w403, y=w404) -> (x-y=w402:dbl[])
          n139 = Divide(x=w410, y=2.0) -> (x/y=w407:dbl[])
          n140 = call "XYtoRPHI.vi"("X-Y"=w402) -> ("r-phi"=w408:dbl[])
          n141 = Index Array(array=w408, index=1) -> (element=w396:dbl)
          n142 = Absolute Value(x=w396) -> (abs(x)=w399:dbl)
          n143 = Sign(1:w396) -> (0:w397:dbl)
          n144 = Subtract(x=w399, y=1.5707963267948966) -> (x-y=w398:dbl)
          n145 = Multiply(x=w397, y=w398) -> (x*y=w395:dbl)
          n146 = Replace Array Subset(array=w407, new element=w395, index=3) -> (w401:dbl[])
        }
        "Measured PickupTool position" <- w375
      }
      event "Deposit Glue": Value Change {
        # "glue box (half-width, half-length, lines)"
        # "Sensor glue pattern Sensor A then B"
        # "Unmount syringe"
        # "first needle park position\nneedle gap on Z value : 0.5 mm"
        # "Syringe-camera offset"
        n147 = event-data() -> ()  [unwired: 1 in, 6 out]
        n148 = call-poly <vilib>:"Read Delimited Spreadsheet.vi"("file path (dialog if empty)"=path "D:/INTT/V1/Assembly Data/Tool Offsets/Dispense Tip Offset.txt", "number of rows (all:-1)"=-1) -> ("first row"=w465:dbl[])  [unwired: 8 in, 5 out]
        n149 = Build Array(11.75, -22, 0.5 ("element"), 0.0 ("element")) -> (w458:dbl[])
        n150 = Index Array(array=w465, index #1=0 ("index"), index #2=1 ("index")) -> (element #1=w460:dbl, element #2=w457:dbl)
        n151 = Build Array(w460, w457, 0.0 ("element"), 0.0 ("element")) -> (w438:dbl[])
        n152 = Add(x=w438, y=w458) -> (x+y=w425:dbl[])
        n153 = Add(x=w426, y=w425) -> (x+y=w444:dbl[])
        "Needle parking position" <- w444
        n154 = call "XYZTheta Go.vi"("XYZTheta In"=w444, "Motion in"=w445) -> ("error out"=w456:errorcluster, "XYZTheta Out"=w454:dbl[], "Motion out"=w443:refnum<class "Motion.lvclass">)  [unwired: 7 in]
        n155 = call "Display Message to User"("error in (no error)"=w456) -> ("error out"=w446:errorcluster)  [unwired: 9 in, 1 out]
        n156 = Select(t=dbl[][] [[-8.43, -62.0, 4.0, 4.0], [-5.62, -59.0, 4.0, 4.0], [-2.81, -56.0, 4.0, 4.0], [0.0, -53.0, 1.0, 1.0], [-8.43, -48.0, 4.0, 0.0], [-5.62, -45.0, 4.0, 0.0], [-2.81, -42.0, 4.0, 0.0], [0.0, -39.0, 1.0, 0.0]], s=w420, f=dbl[][] [[-8.43, -48.0, 4.0, 4.0], [-5.62, -45.0, 4.0, 4.0], [-2.81, -42.0, 4.0, 4.0], [0.0, -39.0, 1.0, 1.0], [-8.43, -62.0, 4.0, 0.0], [-5.62, -59.0, 4.0, 0.0], [-2.81, -56.0, 4.0, 0.0], [0.0, -53.0, 1.0, 0.0]]) -> (s? t:f=w417:dbl[][])
        n157 = Index Array(array=w454, index=2) -> (element=w450:dbl)
        n158 = call-dynamic "Z Go.vi"("error in (no error)"=w446, "Speed"=20.0, "Position"=0.0, "Motion in"=w443) -> ("error out"=w442:errorcluster, "Motion out"=w449:refnum<class "Motion.lvclass">)  [unwired: 6 in]
        n159 = call "Display Message to User2"("error in (no error)"=w442) -> ("error out"=w441:errorcluster)  [unwired: 9 in, 1 out]
        n160 = Add(x=w450, y=-2.5) -> (x+y=w451:dbl)
        n161 = call-dynamic "Z Go.vi"("error in (no error)"=w441, "Speed"=20.0, "Position"=w451, "Motion in"=w449) -> ("error out"=w439:errorcluster, "Motion out"=w440:refnum<class "Motion.lvclass">)  [unwired: 6 in]
        n162 = call-dynamic "Connect.vi"("Ultimus V in"=refnum<class "Ultimus V2.lvclass"> refnum ("Ultimus V2.lvclass")) -> ("Ultimus V out"=w437:refnum<class "Ultimus V2.lvclass">)  [unwired: 9 in, 1 out]
        n163 = case shown="True" w429 {
          tunnel: w440 -> [w481 w584]
          tunnel: w439 -> [w482 w583]
          tunnel: [w480 w582] -> w434
          tunnel: [w482 w581] -> w432
          tunnel: w428 -> [w477 w575]
          tunnel: w438 -> [w476 w580]
          tunnel: w437 -> [w478 w579]
          tunnel: [w479 w578] -> w435
          tunnel: w427 -> [w475 w577]
          tunnel: w417 -> [w474 _]
          tunnel: "Needle Height Compenstation\n(glue gap)" -> [w473 w576]
          tunnel: "check height?" -> [w472 w573]
          tunnel: "Ultimus Pressure" -> [w471 w572]
          frame False {
            # "two sensor, Sensor B then A"
            n164 = for {
              N: w475 -> [_]
              tunnel: w481 -> [w499]
              tunnel: [w498] -> w479
              tunnel: [w497] -> w480
              tunnel: w478 -> [w496]
              tunnel: w477 -> [w495] mode=indexing
              tunnel: w476 -> [w489]
              tunnel: w474 -> [w491]
              tunnel: w473 -> [w485]
              tunnel: w472 -> [w484]
              tunnel: w471 -> [w483]
              i -> [w487]
              # "four\nloops"
              n165 = Multiply(x=4, y=w487) -> (x*y=w486:i32)
              n166 = Array Subset(array=w491, index (row)=w486, length (row)=4 ("length"), index (col)=0, length (col)=3 ("length")) -> (w490:dbl[][])
              "GlueBox" <- w490
              n167 = for {
                N: 4 -> [_]
                tunnel: w499 -> [w559]
                tunnel: [w551] -> w498
                tunnel: [w546] -> w497
                tunnel: w496 -> [w538]
                tunnel: w495 -> [w516]
                tunnel: w490 -> [w513] mode=indexing
                tunnel: w489 -> [w519]
                tunnel: w485 -> [w505]
                tunnel: w484 -> [w502]
                tunnel: w483 -> [w501]
                n168 = Index Array(array=w513, index=0) -> (element=w535:dbl)
                n169 = Index Array(array=w513, index=1) -> (element=w534:dbl)
                n170 = Array Subset(array=w516, index=0, length=2) -> (w518:dbl[])
                n171 = Add(x=w518, y=w519) -> (x+y=w517:dbl[])
                n172 = Absolute Value(x=w535) -> (abs(x)=w533:dbl)
                n173 = Absolute Value(x=w534) -> (abs(x)=w531:dbl)
                n174 = Add(x=w517, y=w513) -> (x+y=w528:dbl[])
                n175 = Multiply(x=w531, y=2.0) -> (x*y=w509:dbl)
                n176 = Multiply(x=w533, y=2.0) -> (x*y=w510:dbl)
                n177 = Multiply(x=w509, y=-1.0) -> (x*y=w521:dbl)
                n178 = Build Array(0.0 ("element"), w509) -> (w529:dbl[])
                n179 = Build Array(w510, 0.0 ("element")) -> (w526:dbl[])
                n180 = Build Array(0.0 ("element"), w521) -> (w507:dbl[])
                n181 = Add(x=w528, y=w529) -> (x+y=w525:dbl[])
                n182 = Add(x=w525, y=w526) -> (x+y=w508:dbl[])
                n183 = call-dynamic "XY Go.vi"("Speed"=200.0, "XY"=w528, "Motion in"=w559) -> ("error out"=w511:errorcluster, "Motion out"=w558:refnum<class "Motion.lvclass">)  [unwired: 7 in]
                n184 = Add(x=w508, y=w507) -> (x+y=w506:dbl[])
                n185 = Index Array(array=w516, index=2) -> (element=w515:dbl)
                n186 = Index Array(array=w513, index=2) -> (element=w512:dbl)
                n187 = Add(x=w515, y=w505) -> (x+y=w544:dbl)
                n188 = Build Array(w525, w508, w506, w528) -> (w520:dbl[][])
                "appended array" <- w520
                n189 = call-dynamic "Z Go.vi"("error in (no error)"=w511, "Speed"=5.0, "Position"=w544, "Motion in"=w558) -> ("error out"=w504:errorcluster, "Motion out"=w554:refnum<class "Motion.lvclass">)  [unwired: 6 in]
                n190 = case shown="True" w502 {
                  tunnel: w504 -> [w563 w565]
                  tunnel: [w563 w564] -> w503
                  frame False {
                  }
                  frame True {
                    n191 = call "Display Message to User11"("error in (no error)"=w565) -> ("error out"=w564:errorcluster)  [unwired: 9 in, 1 out]
                  }
                }
                n192 = call "vacuum.vi"("error in (no error)"=w503, "Vacuum Setting (0000)"=i64 100, "Ultimus V in"=w538) -> ("error out"=w556:errorcluster, "Ultimus V out"=w541:refnum<class "Ultimus V2.lvclass">)  [unwired: 7 in]
                n193 = call-dynamic "Pressure.vi"("error in (no error)"=w556, "Pressure"=w501, "Ultimus V in"=w541) -> ("error out"=w557:errorcluster, "Ultimus V out"=w540:refnum<class "Ultimus V2.lvclass">)  [unwired: 7 in]
                n194 = call-dynamic "Dispense.vi"("error in (no error)"=w557, "Ultimus V in"=w540) -> ("error out"=w553:errorcluster, "Ultimus V out"=w539:refnum<class "Ultimus V2.lvclass">)  [unwired: 8 in]
                n195 = for {
                  N: w512 -> [_]
                  tunnel: w554 -> [w571]
                  tunnel: w553 -> [w570]
                  tunnel: [w569] -> w552
                  tunnel: [w568] -> w550
                  tunnel: w520 -> [w567] mode=indexing
                  (unwired) 4.5 ("Speed")
                  n196 = call-dynamic "XY Go.vi"("error in (no error)"=w570, "Speed"=4.5, "XY"=w567, "Motion in"=w571) -> ("error out"=w569:errorcluster, "Motion out"=w568:refnum<class "Motion.lvclass">)  [unwired: 6 in]
                }
                n197 = Add(x=w544, y=-2.0) -> (x+y=w547:dbl)
                n198 = call-dynamic "Dispense.vi"("error in (no error)"=w552, "Ultimus V in"=w539) -> ("error out"=w545:errorcluster, "Ultimus V out"=w551:refnum<class "Ultimus V2.lvclass">)  [unwired: 8 in]
                n199 = call-dynamic "Z Go.vi"("error in (no error)"=w545, "Speed"=10.0, "Position"=w547, "Motion in"=w550) -> ("Motion out"=w546:refnum<class "Motion.lvclass">)  [unwired: 6 in, 1 out]
              }
            }
          }
          frame True {
            n200 = case shown="True" w573 {
              tunnel: w575 -> [w585 w589]
              tunnel: [w585 w586] -> w574
              frame False {
              }
              frame True {
                n201 = Array Subset(array=w589, index (row)=12 ("index"), length (row)=4 ("length")) -> (w586:dbl[][])  [unwired: 2 in]
              }
            }
            n202 = for {
              N: w577 -> [_]
              tunnel: w584 -> [w633]
              tunnel: w583 -> [w632]
              tunnel: [w622] -> w578
              tunnel: [w621] -> w582
              tunnel: [w620] -> w581
              tunnel: w574 -> [w608] mode=indexing
              tunnel: w580 -> [w607]
              tunnel: w579 -> [w606]
              tunnel: w576 -> [w604]
              tunnel: w573 -> [w601]
              tunnel: w572 -> [_]
              shift-right: [w595] -> _
              shift-left: _ -> [w594]
              i -> [w592]
              # "move the glue in x-dir\n0.1 mm closer to center"
              n203 = Quotient & Remainder(x=w592, y="glue deposit group") -> (x-y*floor(x/y)=w593:i32)  [unwired: 1 out]
              n204 = Equal To 0?(x=w593) -> (x = 0?=w600:bool)
              n205 = Index Array(array=w608, index=2) -> (element=w609:dbl)
              n206 = Add(x=w608, y=w607) -> (x+y=w631:dbl[])
              n207 = Build Array(0.0 ("element"), 3.3 ("element")) -> (w636:dbl[])
              n208 = Subtract(x=w631, y=w636) -> (x-y=w637:dbl[])
              n209 = Add(x=w609, y=w604) -> (x+y=w610:dbl)
              n210 = Add(x=w631, y=w636) -> (x+y=w618:dbl[])
              n211 = call-dynamic "XY Go.vi"("error in (no error)"=w632, "Speed"=200.0, "XY"=w637, "Motion in"=w633) -> ("error out"=w623:errorcluster, "Motion out"=w616:refnum<class "Motion.lvclass">)  [unwired: 6 in]
              n212 = call-dynamic "Z Go.vi"("error in (no error)"=w623, "Speed"=5.0, "Position"=w610, "Motion in"=w616) -> ("error out"=w603:errorcluster)  [unwired: 6 in, 1 out]
              n213 = case shown="True" w601 {
                tunnel: w603 -> [w660 w662]
                tunnel: [w660 w661] -> w602
                frame False {
                }
                frame True {
                  n214 = call "Display Message to User7"("error in (no error)"=w662) -> ("error out"=w661:errorcluster)  [unwired: 9 in, 1 out]
                }
              }
              n215 = call "vacuum.vi"("error in (no error)"=w602, "Vacuum Setting (0000)"=i64 100, "Ultimus V in"=w606) -> ("error out"=w596:errorcluster, "Ultimus V out"=w597:refnum<class "Ultimus V2.lvclass">)  [unwired: 7 in]
              n216 = case shown="True" w600 {
                tunnel: [w639 w651] -> w599
                tunnel: [w640 w650] -> w598
                tunnel: w597 -> [w642 w649]
                tunnel: w596 -> [w641 w647]
                tunnel: [w638 w644] -> w595
                tunnel: w594 -> [w638 _]
                tunnel: [w638 w643] -> w590
                frame False {
                  n217 = call-dynamic "Pressure.vi"("error in (no error)"=w641, "Pressure"=w638, "Ultimus V in"=w642) -> ("error out"=w639:errorcluster, "Ultimus V out"=w640:refnum<class "Ultimus V2.lvclass">)  [unwired: 7 in]
                }
                frame True {
                  n218 = flat-sequence {
                    tunnel: [w654] -> _
                    tunnel: w649 -> [w654]
                    tunnel: [w654] -> w648
                    tunnel: w647 -> [w653]
                    tunnel: [w653] -> w646
                    tunnel: [w652] -> w645
                    tunnel: [w652] -> w644
                    tunnel: [w659] -> w651
                    tunnel: [w658] -> w650
                    tunnel: w648 -> [w657]
                    tunnel: w646 -> [w656]
                    tunnel: w645 -> [w655]
                    tunnel: [w655] -> w643
                    frame #0 {
                      n219 = call "air pressure setting.vi"() -> ("air pressure indecator"=w652:i32)  [unwired: 1 out]
                    }
                    frame #1 {
                      n220 = call-dynamic "Pressure.vi"("error in (no error)"=w656, "Pressure"=w655, "Ultimus V in"=w657) -> ("error out"=w659:errorcluster, "Ultimus V out"=w658:refnum<class "Ultimus V2.lvclass">)  [unwired: 7 in]
                    }
                  }
                }
              }
              "air pressure indecator" <- w590
              n221 = call-dynamic "Dispense.vi"("error in (no error)"=w599, "Ultimus V in"=w598) -> ("error out"=w617:errorcluster, "Ultimus V out"=w624:refnum<class "Ultimus V2.lvclass">)  [unwired: 8 in]
              n222 = call "Time Delay"("error in (no error)"=w617) -> ("error out"=w615:errorcluster)  [unwired: 10 in]
              n223 = call-dynamic "XY Go.vi"("error in (no error)"=w615, "Speed"=5.0, "XY"=w618, "Motion in"=w616) -> ("error out"=w614:errorcluster, "Motion out"=w612:refnum<class "Motion.lvclass">)  [unwired: 6 in]
              n224 = call "Time Delay3"("error in (no error)"=w614) -> ("error out"=w613:errorcluster)  [unwired: 10 in]
              n225 = call "Time Delay2"("error in (no error)"=w615) -> ("error out"=w625:errorcluster)  [unwired: 10 in]
              n226 = call-dynamic "Dispense.vi"("error in (no error)"=w625, "Ultimus V in"=w624) -> ("Ultimus V out"=w622:refnum<class "Ultimus V2.lvclass">)  [unwired: 8 in, 1 out]
              n227 = Add(x=w610, y=-2.5) -> (x+y=w628:dbl)
              n228 = call-dynamic "Z Go.vi"("error in (no error)"=w613, "Speed"=10.0, "Position"=w628, "Motion in"=w612) -> ("error out"=w620:errorcluster, "Motion out"=w621:refnum<class "Motion.lvclass">)  [unwired: 6 in]
            }
          }
        }
        n229 = call-dynamic "Disconnect.vi"("Ultimus V in"=w435) -> ()  [unwired: 9 in, 1 out]
        n230 = call "XYZTheta Go.vi"("error in (no error)"=w432, "XYZTheta In"=dbl[] [400.0, 600.0, 0.0, 0.1], "Motion in"=w434) -> ("error out"=w433:errorcluster, "Motion out"=w430:refnum<class "Motion.lvclass">)  [unwired: 6 in, 1 out]
        n231 = call "Display Message to User3"("error in (no error)"=w433) -> ()  [unwired: 9 in, 2 out]
      }
      event "Needle Alignment": Value Change {
        (unwired) "Needle Alignment in progress ...." ("String")
        # "first needle park position\nneedle gap on Z value : 0.5 mm"
        # "Syringe-camera offset"
        n232 = event-data() -> ()  [unwired: 1 in, 6 out]
        n233 = call-poly <vilib>:"Read Delimited Spreadsheet.vi"("file path (dialog if empty)"=path "D:/INTT/V1/Assembly Data/Tool Offsets/Dispense Tip Offset.txt", "number of rows (all:-1)"=-1) -> ("first row"=w704:dbl[])  [unwired: 8 in, 5 out]
        n234 = Build Array(11.75, -25, 0.5 ("element"), 0.0 ("element")) -> (w697:dbl[])
        n235 = Index Array(array=w704, index #1=0 ("index"), index #2=1 ("index")) -> (element #1=w699:dbl, element #2=w696:dbl)
        n236 = Build Array(w699, w696, 0.0 ("element"), 0.0 ("element")) -> (w666:dbl[])
        n237 = Add(x=w666, y=w697) -> (x+y=w690:dbl[])
        n238 = Add(x=w689, y=w690) -> (x+y=w691:dbl[])
        n239 = call "XYZTheta Go.vi"("XYZTheta In"=w691, "Motion in"=w681) -> ("error out"=w695:errorcluster, "XYZTheta Out"=w671:dbl[], "Motion out"=w680:refnum<class "Motion.lvclass">)  [unwired: 7 in]
        n240 = call "Display Message to User10"("error in (no error)"=w695) -> ("error out"=w692:errorcluster)  [unwired: 9 in, 1 out]
        n241 = call-dynamic "Z Go.vi"("error in (no error)"=w692, "Speed"=20.0, "Position"=0.0, "Motion in"=w680) -> ("Motion out"=w679:refnum<class "Motion.lvclass">)  [unwired: 6 in, 1 out]
        n242 = Replace Array Subset(array=w671, new element=0.0 ("new element/subarray"), index=2) -> (w668:dbl[])
        n243 = call "Joystick and Camera SHIH VPC- external Connection.vi"("Motion in"=w679, "XYZTheta"=w668, "Measurement Point"="Touch Needle on a surface") -> ("Motion out"=w677:refnum<class "Motion.lvclass">, "Gantry"=w667:dbl[])  [unwired: 4 in, 2 out]
        n244 = Subtract(x=w667, y=w666) -> (x-y=w665:dbl[])
        n245 = call "Joystick and Camera SHIH VPC- external Connection.vi"("Motion in"=w677, "XYZTheta"=w665, "Measurement Point"="Measure the touch spot with camera") -> ("Motion out"=w673:refnum<class "Motion.lvclass">, "Gantry"=w676:dbl[])  [unwired: 4 in, 2 out]
        n246 = Subtract(x=w667, y=w676) -> (x-y=w675:dbl[])
        n247 = call-poly <vilib>:"Write Delimited Spreadsheet.vi"("file path (dialog if empty)"=path "D:/INTT/V1/Assembly Data/Tool Offsets/Dispense Tip Offset.txt", "1D data"=w675, "append to file? (new file:F)"=FALSE) -> ()  [unwired: 11 in, 2 out]
      }
      event "Pick and place": Value Change {
        (unwired) "PICK and PLACE samples ..." ("String")
        (unwired) -21.3804 ("new element/subarray")
        n248 = event-data() -> ()  [unwired: 1 in, 6 out]
        n249 = call-poly <vilib>:"Read Delimited Spreadsheet.vi"("file path (dialog if empty)"=path "D:/INTT/V1/Assembly Data/Tool Offsets/Bellows Tool Offset.txt", "number of rows (all:-1)"=-1) -> ("first row"=w734:dbl[])  [unwired: 8 in, 5 out]
        n250 = Select(t=1, s=w711, f=w723) -> (s? t:f=w739:i32)
        n251 = Index Array(array=w734, index #1=0 ("index"), index #2=1 ("index"), index #3=2 ("index")) -> (element #1=w730:dbl, element #2=w729:dbl, element #3=w728:dbl)
        n252 = case shown="True" w719 {
          tunnel: [w740 w743] -> w718
          tunnel: w713 -> [w740 w742]
          frame False {
          }
          frame True {
            # "sensor A"
            # "sensor B"
            n253 = Index Array(array=w742, index=0) -> (element=w741:i32)
            n254 = Index Array(array=w742, index=1) -> (element=w744:i32)
            n255 = Build Array(w744, w741) -> (w743:i32[])
          }
        }
        n256 = for {
          N: w739 -> [_]
          tunnel: w723 -> [w783]
          tunnel: w724 -> [w779]
          tunnel: w737 -> [w803]
          tunnel: [w791] -> w727
          tunnel: w725 -> [w801] mode=indexing
          tunnel: [w767] -> w717
          tunnel: w716 -> [w754]
          tunnel: w730 -> [w793]
          tunnel: w729 -> [w792]
          tunnel: w726 -> [w776]
          tunnel: w728 -> [w790]
          tunnel: w711 -> [w760]
          tunnel: w718 -> [w748] mode=indexing
          tunnel: "VacChannel for sample" -> [w762]
          tunnel: "check height? 2" -> [w755]
          tunnel: w711 -> [w747]
          i -> [w769]
          w752 = 0 ("Channel")
          w751 = TRUE ("Value")
          # "put back pickup tool"
          # "if chips, do one pickup tool and multiple samples;\nif sensors, one pickup tool for one sample ( so 2->2);"
          # "build a fake 2d arrays"
          # "sensor"
          # "chip pickup tool"
          # "pickup tool height offset"
          # "Pick up PICKUP TOOL"
          # "Pick up CHIPs/Sensor and place on HDI"
          n257 = Select(t=w783, s=w760, f=1) -> (s? t:f=w782:i32)
          n258 = Build Array(w793, w792, w790, 0.0 ("element")) -> (w788:dbl[])
          n259 = Add(x=w801, y=w788) -> (x+y=w789:dbl[])
          n260 = call "XYZTheta-2Zspeed Go.vi"("XYZTheta In"=w789, "Motion in"=w803) -> ("error out"=w750:errorcluster, "Motion out"=w802:refnum<class "Motion.lvclass">)  [unwired: 7 in, 1 out]
          n261 = Select(t=-18.52 ("new element/subarray"), s=w760, f=-13.13 ("t")) -> (s? t:f=w784:dbl)
          n262 = call "WriteReadWait.vi"("Read Value"=w751, "Write Value"=w751, "error in (no error)"=w750, "Read"=w752, "Write"=w752, "I-O in"=w754) -> ("error out"=w749:errorcluster, "I-O out"=w753:refnum<class "NI-DAQ.lvclass">)  [unwired: 4 in]
          n263 = Replace Array Subset(array=w788, new element=w784, index=2) -> (w786:dbl[])
          n264 = Index Array(array=w779, index (row)=w769) -> (element=w778:dbl[])  [unwired: 1 in]
          n265 = call "Time Delay8"("error in (no error)"=w749) -> ("error out"=w799:errorcluster)  [unwired: 10 in]
          n266 = Build Array(w778, w778) -> (w777:dbl[][])
          n267 = Select(t=w779, s=w760, f=w777) -> (s? t:f=w780:dbl[][])
          n268 = Index Array(array=w776, index (row)=w769) -> (element=w775:dbl[])  [unwired: 1 in]
          n269 = Build Array(w775, w775) -> (w774:dbl[][])
          n270 = Select(t=w776, s=w760, f=w774) -> (s? t:f=w757:dbl[][])
          n271 = case shown="True" w755 {
            tunnel: [w804 w806] -> w756
            tunnel: w757 -> [w804 w805]
            frame False {
            }
            frame True {
              n272 = Array Subset(array=w805, index (row)=12 ("index"), length (row)=4 ("length")) -> (w806:dbl[][])  [unwired: 2 in]
            }
          }
          n273 = Select(t="chip placement height compensation", s=w760, f=0.0) -> (s? t:f=w758:dbl)
          n274 = for {
            N: w782 -> [_]
            tunnel: w780 -> [w823] mode=indexing
            tunnel: w802 -> [w825]
            tunnel: w786 -> [w824]
            tunnel: w799 -> [w822]
            tunnel: [w821] -> w794
            tunnel: w753 -> [w820]
            tunnel: w756 -> [w817] mode=indexing
            tunnel: [w816] -> w785
            tunnel: w758 -> [w815]
            tunnel: w748 -> [w814]
            tunnel: w762 -> [w813]
            tunnel: [w812] -> w761
            tunnel: w760 -> [w811]
            tunnel: w755 -> [w810]
            tunnel: w747 -> [w809]
            n275 = flat-sequence {
              tunnel: w823 -> [w842]
              tunnel: [w844] -> w826
              tunnel: w825 -> [w843]
              tunnel: w824 -> [w841]
              tunnel: w822 -> [w839]
              tunnel: w820 -> [w837]
              tunnel: [w831] -> w819
              tunnel: [w832] -> w818
              tunnel: w814 -> [w834]
              tunnel: w813 -> [w829]
              tunnel: w826 -> [w867]
              tunnel: [w866] -> w821
              tunnel: w824 -> [w864]
              tunnel: w819 -> [w865]
              tunnel: w818 -> [w852]
              tunnel: w817 -> [w863]
              tunnel: [w846] -> w816
              tunnel: w815 -> [w856]
              tunnel: w813 -> [w851]
              tunnel: [w847] -> w812
              tunnel: w811 -> [_]
              tunnel: w810 -> [w853]
              tunnel: w809 -> [w845]
              frame #0 {
                w830 = TRUE ("Value")
                w833 = FALSE ("Value")
                # "pickup sample"
                # "release sample from tray"
                # "pickup sample from tray"
                n276 = Add(x=w842, y=w841) -> (x+y=w840:dbl[])
                n277 = call "XYZTheta-2Zspeed Go.vi"("error in (no error)"=w839, "XYZTheta In"=w840, "Motion in"=w843) -> ("error out"=w838:errorcluster, "Motion out"=w844:refnum<class "Motion.lvclass">)  [unwired: 6 in, 1 out]
                n278 = call "Time Delay4"("error in (no error)"=w838) -> ("error out"=w835:errorcluster)  [unwired: 10 in]
                n279 = call "WriteReadWait.vi"("Read Value"=w833, "Write Value"=w833, "error in (no error)"=w835, "Read"=w834, "Write"=w834, "I-O in"=w837) -> ("error out"=w836:errorcluster, "I-O out"=w828:refnum<class "NI-DAQ.lvclass">)  [unwired: 4 in]
                n280 = call "Time Delay11"("error in (no error)"=w836) -> ("error out"=w827:errorcluster)  [unwired: 10 in]
                n281 = call "WriteReadWait.vi"("Read Value"=w830, "Write Value"=w830, "error in (no error)"=w827, "Read"=w829, "Write"=w829, "I-O in"=w828) -> ("error out"=w831:errorcluster, "I-O out"=w832:refnum<class "NI-DAQ.lvclass">)  [unwired: 4 in]
              }
              frame #1 {
                w849 = FALSE ("Value")
                # "release sample on HDI"
                # "lift for chip/sensor thickness"
                # "place sample on HDI"
                n282 = Add(x=w863, y=w864) -> (x+y=w859:dbl[])
                n283 = Build Array(0.0 ("element"), 0.0 ("element"), w856, 0.0 ("element")) -> (w858:dbl[])
                n284 = Add(x=w859, y=w858) -> (x+y=w857:dbl[])
                n285 = call "XYZTheta-2Zspeed Go.vi"("error in (no error)"=w865, "XYZTheta In"=w857, "Motion in"=w867) -> ("error out"=w855:errorcluster, "Motion out"=w866:refnum<class "Motion.lvclass">)  [unwired: 6 in, 1 out]
                n286 = case shown="True" w853 {
                  tunnel: w855 -> [w872 w874]
                  tunnel: [w872 w873] -> w854
                  frame False {
                  }
                  frame True {
                    n287 = call "Display Message to User6"("error in (no error)"=w874) -> ("error out"=w873:errorcluster)  [unwired: 9 in, 1 out]
                  }
                }
                n288 = case shown="True" w845 {
                  tunnel: w854 -> [w869 w871]
                  tunnel: [w868 w870] -> w850
                  frame False {
                    n289 = call "Time Delay7"("error in (no error)"=w869) -> ("error out"=w868:errorcluster)  [unwired: 10 in]
                  }
                  frame True {
                    n290 = call "Time Delay6"("error in (no error)"=w871) -> ("error out"=w870:errorcluster)  [unwired: 10 in]
                  }
                }
                n291 = call "WriteReadWait.vi"("Read Value"=w849, "Write Value"=w849, "error in (no error)"=w850, "Read"=w851, "Write"=w851, "I-O in"=w852) -> ("error out"=w848:errorcluster, "I-O out"=w847:refnum<class "NI-DAQ.lvclass">)  [unwired: 4 in]
                n292 = call "Time Delay5"("error in (no error)"=w848) -> ("error out"=w846:errorcluster)  [unwired: 10 in]
              }
            }
          }
          n293 = call "XYZTheta-2Zspeed Go.vi"("error in (no error)"=w785, "XYZTheta In"=w789, "Motion in"=w794) -> ("error out"=w759:errorcluster, "Motion out"=w798:refnum<class "Motion.lvclass">)  [unwired: 6 in, 1 out]
          n294 = call "Time Delay9"("error in (no error)"=w759) -> ("error out"=w765:errorcluster)  [unwired: 10 in]
          n295 = call-dynamic "Digital Write 1 Channel.vi"("DAQ Module"=0, "error constant"=w765, "Value"=FALSE, "Channel"=0, "NI-DAQ.lvclass"=w761) -> ("error IO"=w768:errorcluster, "NI-DAQ.lvclass 2"=w767:refnum<class "NI-DAQ.lvclass">)  [unwired: 5 in]
          n296 = call "Time Delay10"("error in (no error)"=w768) -> ("error out"=w795:errorcluster)  [unwired: 10 in]
          n297 = call-dynamic "Z Go.vi"("error in (no error)"=w795, "Speed"=20.0, "Position"=0.0 ("new element/subarray"), "Motion in"=w798) -> ("Motion out"=w791:refnum<class "Motion.lvclass">)  [unwired: 6 in, 1 out]
        }
      }
      event "GOTO": Value Change {
        (unwired) "GOING to a position" ("String")
        n298 = event-data() -> ()  [unwired: 1 in, 6 out]
        n299 = call "XYZTheta-2Zspeed Go.vi"("XYZTheta In"="Parking position", "Motion in"=w878) -> ("Motion out"=w877:refnum<class "Motion.lvclass">)  [unwired: 7 in, 2 out]
      }
      event "READ Position": Value Change {
        n300 = event-data() -> ()  [unwired: 1 in, 6 out]
        n301 = call-dynamic "Get Current Position.vi"("Motion in"=w900) -> ("XYZTheta Out"=→"Gantry current position":dbl[], "Motion out"=w899:refnum<class "Motion.lvclass">)  [unwired: 8 in, 1 out]
      }
      event "TrayVaccum": Value Change {
        n302 = event-data() -> ()  [unwired: 1 in, 6 out]
        n303 = Index Array(array=w903, index=0) -> (element=w912:i32)
        n304 = Index Array(array="Values", index=0) -> (element=w906:bool)
        n305 = call "WriteReadWait.vi"("Read Value"=w906, "Write Value"=w906, "Read"=w912, "Write"=w912, "I-O in"=w915) -> ("error out"=w911:errorcluster, "I-O out"=w914:refnum<class "NI-DAQ.lvclass">)  [unwired: 5 in]
        n306 = Index Array(array=w903, index=1) -> (element=w909:i32)
        n307 = Index Array(array="Values", index=1) -> (element=w904:bool)
        n308 = call "WriteReadWait.vi"("Read Value"=w904, "Write Value"=w904, "error in (no error)"=w911, "Read"=w909, "Write"=w909, "I-O in"=w914) -> ("I-O out"=w901:refnum<class "NI-DAQ.lvclass">)  [unwired: 4 in, 1 out]
      }
      event Timeout {
        n309 = event-data() -> ()  [unwired: 1 in, 3 out]
        n310 = call-dynamic "Digital Read Multiple Channels.vi"("Array"=w928, "NI-DAQ in"=w927) -> ("subarray"=w929:bool[], "NI-DAQ out"=w925:refnum<class "NI-DAQ.lvclass">)  [unwired: 7 in, 1 out]
      }
    }
    "Measure HDI top-left" <- w36
    "Sample on HDI" <- w8
    "vacuum on?" <- w11
    n311 = feedback-in #1(w34) -> ()
    n312 = feedback-in #2(w36) -> ()
    n313 = feedback-in #3(w31) -> ()
    n314 = feedback-in #4(w23) -> ()
    n315 = feedback-in #5(w20) -> ()
    n316 = feedback-in #6(w11) -> ()
    n317 = feedback-in #7(w28) -> ()
    n318 = feedback-in #8(w8) -> ()
    n319 = feedback-in #9(w29) -> ()
    "# of tasks excuted" <- w25
  }
  n320 = call-dynamic "Disconnect.vi"("I-O in"=w1) -> ()  [unwired: 9 in, 1 out]
  n321 = call-dynamic "Disconnect.vi"("Controller in"=w4) -> ()  [unwired: 9 in, 1 out]
